vi "main.vi"(8 "error in (no error)":errorcluster, 10 "stages":refnum<class "_stage.lvclass">[](array[class]), 11 "_camera":refnum<class "_camera.lvclass">) -> ()   [LabVIEW 2019]
uses:
  _camera/_camera.lvlibp/_cameraClass/_camera.lvclass
  _stage/_stage.lvlibp/_stageClass/_stage.lvclass
  data_algorithm.ctl
  state.ctl
  data_process.ctl
  <vilib>/Analysis/baseanly.llb/Mean (DBL).vi
  378a35e6-17c3-42fc-973f-4dbb75f37032.vi
  972fad81-3ff3-4c5b-b5d6-c93ea4aec52b.vi
  951adbdd-488d-47b0-b06c-8d69e9ccb4aa.vi
  2b97118a-447f-4295-80f1-8ed8751fa7ac.vi
  <vilib>/Utility/config.llb/Read Key (Path).vi
  <vilib>/Utility/config.llb/Read Key (String).vi
  _camera/_camera.lvlibp/_cameraClass/Write stage positions readback.vi
  _camera/_camera.lvlibp/_cameraClass/Write config file path.vi
  _camera/_camera.lvlibp/_cameraClass/Read camera name and version.vi
  _camera/_camera.lvlibp/_cameraClass/Read wavelength.vi
  _camera/_camera.lvlibp/_cameraClass/Write background.vi
  <vilib>/gmath/NumericalOptimization/Nonlinear Curve Fit LM formula string.vi
  _camera/_camera.lvlibp/_cameraClass/Write wavelength.vi
  _camera/_camera.lvlibp/_cameraClass/Read stage positions.vi
  _camera/_camera.lvlibp/_cameraClass/Write stage positions.vi
  <vilib>/Utility/file.llb/Read Delimited Spreadsheet (DBL).vi
  <vilib>/Utility/config.llb/Read Key (Double).vi
  <vilib>/Analysis/NI_AALBase.lvlib
  <vilib>/Utility/config.llb/NI_LVConfig.lvlib
  <vilib>/gmath/NI_Gmath.lvlib
panel:
  out "signal anis. (accum.)":dbl[][](graph)
  in  "FROG wl_min_max":dbl[](array[numeric])
  out "millisecond timer value 2":u32
  out "Boolean 3":bool=TRUE
  out "cont acq. time":u32
  out "millisecond timer value":u32
  out "plot time":u32
  out "data proc.":u32
  in  "indep?":bool[](array[boolean])
  out "scan done?":bool
  in  "FROG?":bool
  out "size of dependent time scan":i32
  out "single acq. time":u32
  out "single loop time":u32=150 caption="usec"
  in  "which plot":u16(ring)=2 items=["pumped", "unpumped", "reference", "difference"]
  in  "Algorithm":T1=3 items=["<(S*-S)/S>/ln(10)", "<S*/S>-1", "<S*/PD*>/<S/PD>", "<S*/Sref*>/<S/Sref>", "<S*/Sref*/PD*>/<S/Sref>", "<S*/Sref*>/<S/Sref>_alt", "MA/r", "MA/r Sagnac", "FROG"]
  in  "show reference spectrum?":bool
  in  "remove cursor":bool
  in  "add cursor":bool
  out "Array":i32[](array[numeric])
  out "x = y?":bool
  in  "reversed?":bool[](array[boolean])=[TRUE]
  in  "Experimenter":string="who are you?"
  in  "Title":string="A clever title"
  in  "Experimental parameters":string="sample:\nsolvent:\ncuvette:\noptical density:\nexcitation wavelength:\nexcitation power:\nexcitation spot size:\nexcitation fluence: \nprobe spot size:\ncomment:"
  out "current scan":i32
  in  "N scans":u16=5
  in  "sample":string="testSample"
  in  "Experiment":string="testExp"
  in  "center cursor":bool
  in  "save flag":bool
  in  "save type":bool[](array[boolean])=[FALSE, FALSE, FALSE, FALSE]
  in  "data folder":path=path "Z:/11 Setups/04 NOPA TA/01 Data"
  out "progress":dbl(slide)=21.0 scale=0.0..100.0
  out "scan progress":u8(slide)=16 scale=0.0..100.0
  out "Cursor position (wl)":dbl[](array[numeric]) format="%#.2g"
  out "Cursor position (idx)":dbl[](array[numeric])
  in  "ampl":cluster{dbl, dbl}(slide)={-0.2917505030181087, 6.9678068410462775} scale=-1.0..10.0
  in  "diff":dbl(slide)=26.28128772635815 scale=0.05..50.0
  out "main graph":cluster{"wavelength":dbl[], "ref mean":dbl[]}[](graph)
  in  "time delay file":path=path "D:/github/TransientAbsorptionDAQ.lv/stepfiles/01_coarseSteps_-1000_1000fs.txt"
  in  "scan":bool
  in  "bottom panel":u16(ring)=2 items=["x/y", "y/x", "traces", "std", "debug", "debug 2", "parameters", "wavelength"]
  in  "parity?":enum32{"Item 0", "Item 1"}(radio)
  out "Camera initialised?":bool[](array[boolean])
  out "Char":i16
  in  "view error anal":bool
  in  "view full data":bool
  in  "get bg":bool
  in  "cont acq":bool
  in  "move stage":enum32{"Item 0", "Item 1"}(radio)
  out "timed out?":bool
  out "Boolean":bool
  out "Stage(s) initialized":bool[](array[boolean])
  in  "set as t0":bool[](array[boolean])
  in  "home stages":bool[](array[boolean])
  out "stage name(s)":i32[](listbox)
  out "Tab Control":T2(tab)
  out "Intensity Chart":dbl[][](graph)
  out "Intensity Graph":dbl[][](graph)
  out "Waveform Chart":T3(graph)
  out "std graph":cluster{"wavelength":dbl[], "ref std":dbl[]}[](graph)
  out "std":dbl
  out "std":dbl
  out "skipped":bool[](array[boolean])
  out "chopper out":bool[][](array[boolean])
  out "synchronization error":bool
  out "mean":dbl
  out "mean":dbl
  out "PD hist":T4(graph)
  out "PD":cluster{i32[], dbl[]}[](graph)
  in  "ts_plot_lin-log":bool caption="timestep_plot_linlog"
  out "base path":path
  out "stage config":path
  out "camera config":path
  out "Application Directory":path
  out "appended path":path
  out "Stage objects":refnum<class "_stage.lvclass">[](array[class])
  out "timesteps loaded from file":dbl[][](array[numeric])
  out "size of dependent time scan 2":i32
  out "Waveform Graph":dbl[](graph)
  in  "trig2 level":dbl(slide)=783.9195979899498 scale=0.0..2000.0
  out "Tank 2":dbl(slide) scale=0.0..2000.0
  out "Tank 2 + std":dbl(slide) scale=0.0..2000.0
  out "Tank 2 - std":dbl(slide) scale=0.0..2000.0
  in  "trig1 level":dbl(slide)=783.9195979899498 scale=0.0..2000.0
  out "Tank 1":dbl(slide)=552.7638190954774 scale=0.0..2000.0
  out "Tank 1 - std":dbl(slide) scale=0.0..2000.0
  out "Tank 1 + std":dbl(slide) scale=0.0..2000.0
  in  "baseline offset (ref.)":dbl
  in  "baseline offset (signal)":dbl
  in  "history length":i32=20
  in  "Scale.Range:Maximum":dbl(slide)=43.976036093027226 caption="diff scale range" scale=1.0..1000.0
  in  "camera max scale":u16(ring) items=["16-bit", "14-bit", "12-bit"]
  in  "save raw data":bool caption="saw raw data"
  in  "is measurement TA?":bool=TRUE
  out "Boolean 2":bool
  out "element 2":dbl
  out "element 3":dbl
  out "PDs mean":dbl[](array[numeric])
  out "PDs std":dbl[](array[numeric])
  out "dynamic offset":dbl[](array[numeric])
  in  "use dynamic offset?":bool
  in  "save wl calibration to .ini":bool caption="calibrate_wl"
  in  "index":u16
  in  "calibrate wavelength":bool caption="calibrate_wl"
  out "wavelength fit":cluster{i32[], dbl[]}[](graph)
  out "wavelength (fitted)":dbl[](array[numeric]) format="%#.0f"
  in  "wavelength \n(calibration value)":dbl[](array[numeric]) caption="wavelength (calibration value)"
  in  "pixel/index":u16[](array[numeric])
  in  "mirror?":bool
  in  "initial parameters":dbl[](array[numeric])=[150.0, 200000.0, 1200.0]
  out "best fit parameters":dbl[](array[numeric])
  in  "t0 position(s)":dbl[](array[numeric]) caption="t0 (s)" format="%07.0f"
  out "stage position(s) readback":dbl[](array[numeric]) caption="readback (fs)" format="%09.1f"
  in  "stage position(s)":dbl[](array[numeric]) caption="set (fs)" format="%09.1f"
  out "camera name, version":string
  in  "get_single_acq":bool caption="get single"
  out "vi running?":bool=TRUE
  out "is moving?":bool[](array[boolean]) caption="mov?"
  # "scan"
  # "out of"
  # "just temp ..."
  # "timing"
  # "usec"
  # "transient"
  # "pumped mean"
  # "unpumped mean"
  # "reference mean"
  # "Hartmann dispersion formula:"
  # "d(\\lambda) = a1 + a2 / (pix - a3)"
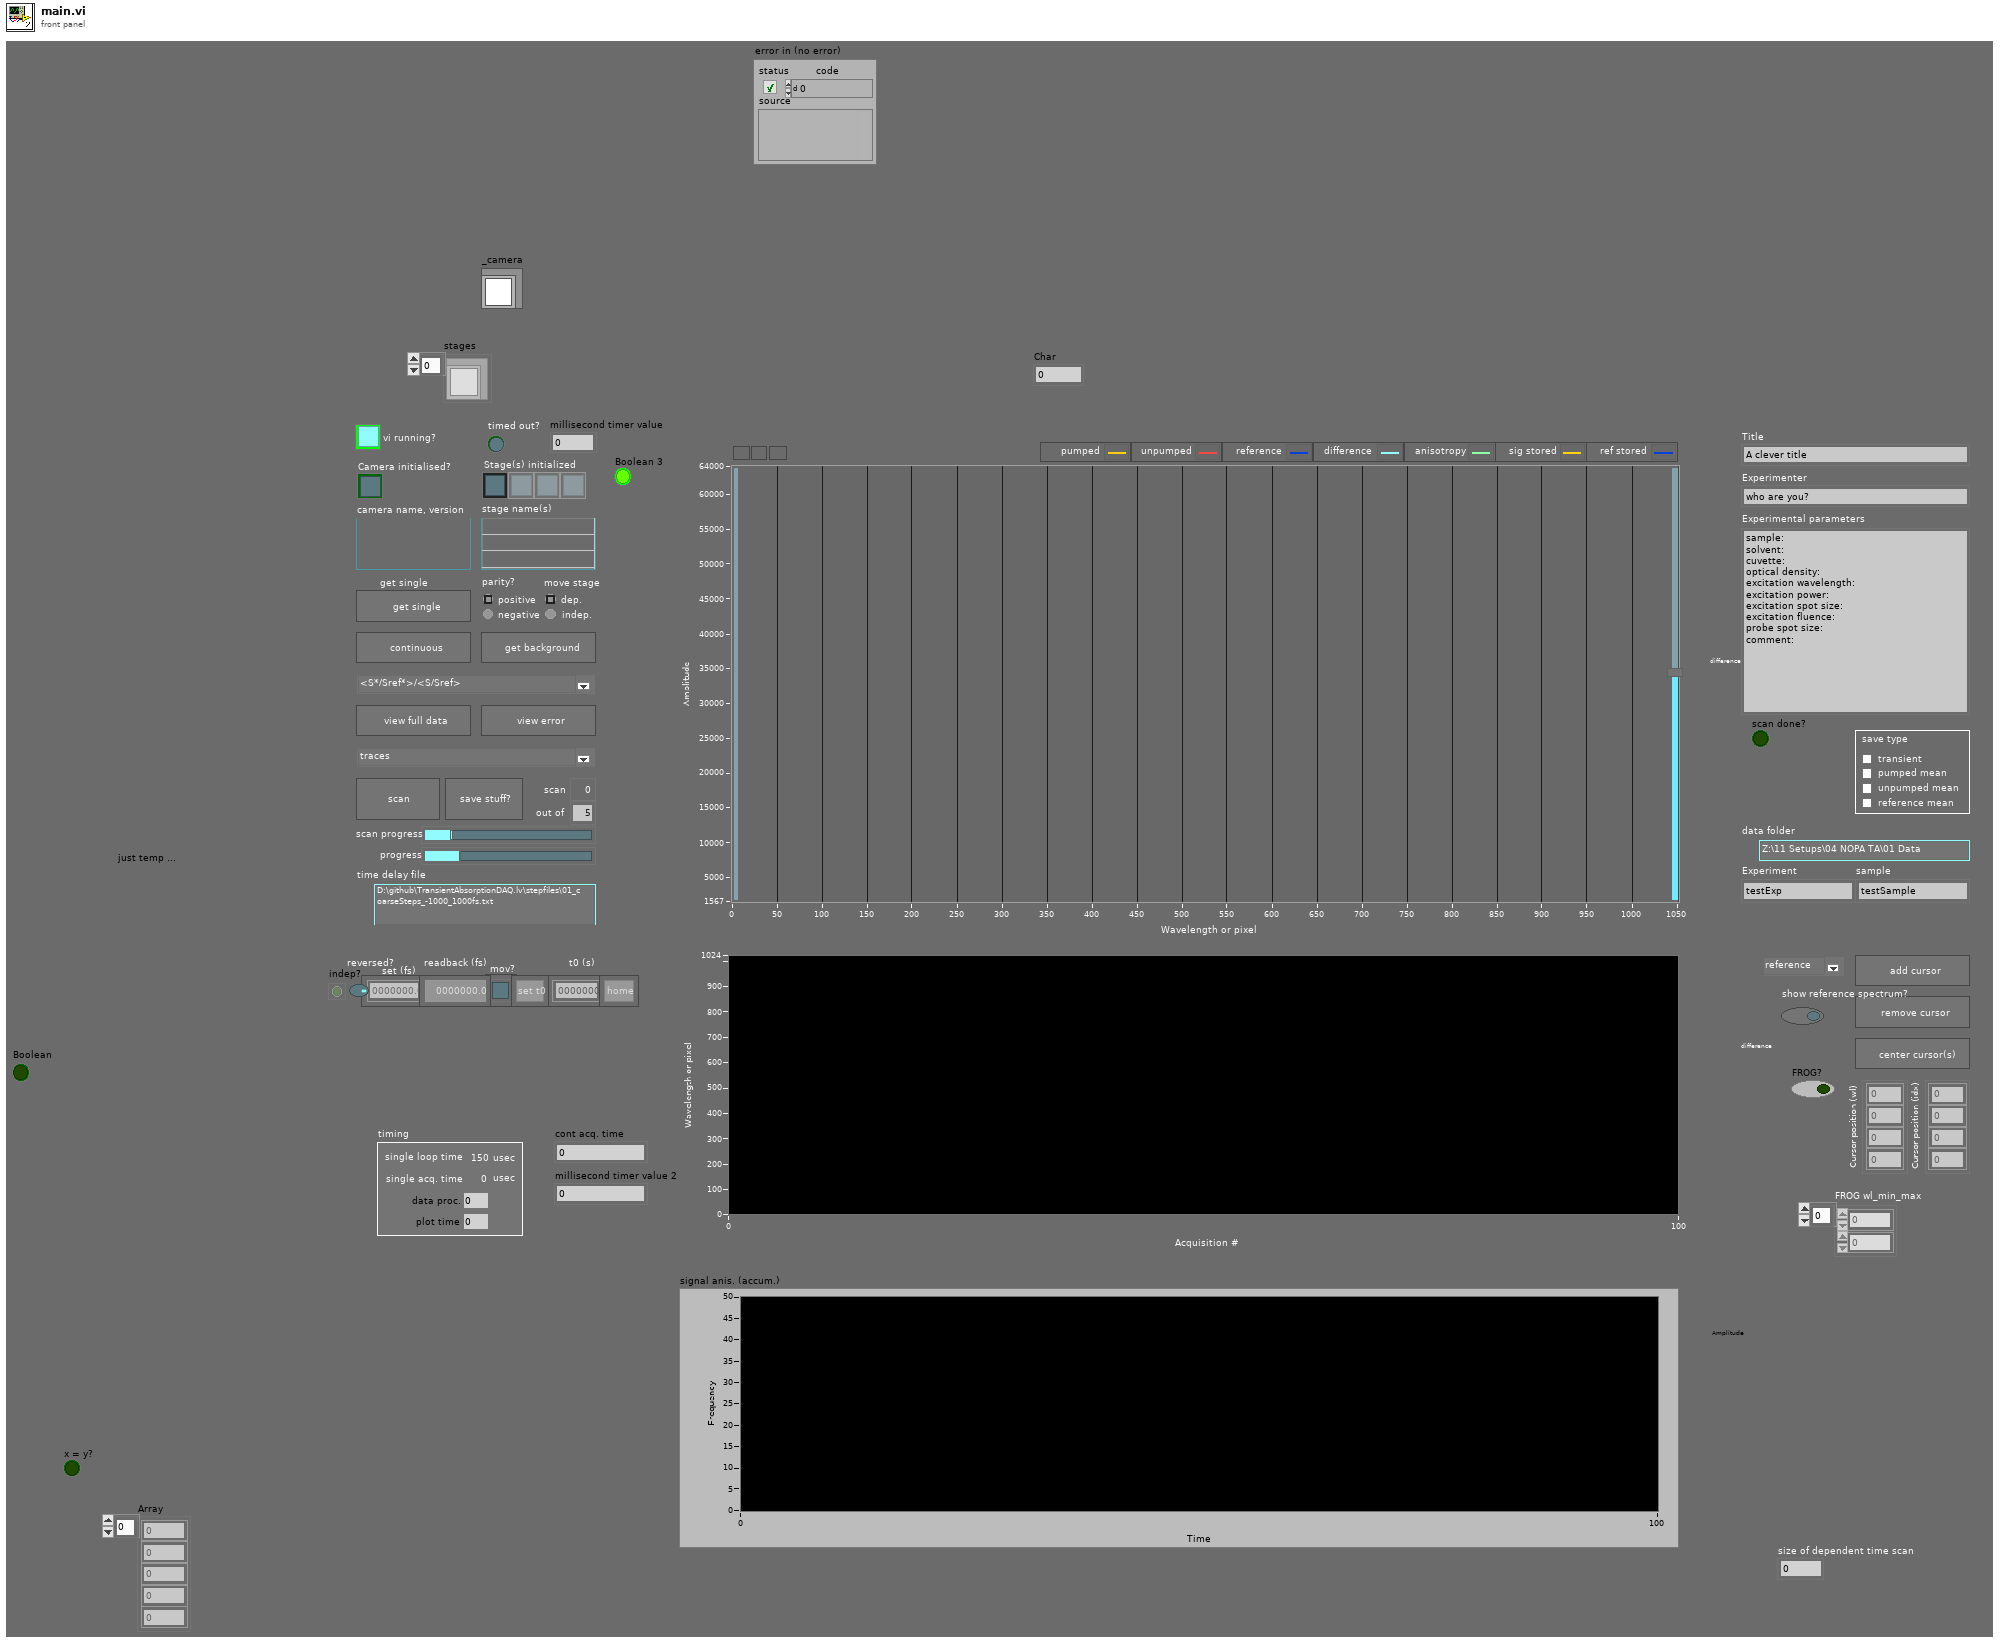
[diagram p1: front panel]
types:
  T1 = typedef "data_algorithm.ctl" = u16
  T2 = enum32{"x/y", "y/x", "traces", "std", "debug", "debug 2", "parameters", "wavelength"}
  T3 = cluster{"[0]":dbl, "[1]":dbl, "[2]":dbl, "[3]":dbl, "[4]":dbl, "[5]":dbl, "[6]":dbl, "[7]":dbl, "[8]":dbl}
  T4 = cluster{"Histogram: h(x)":i32[], "X Values":dbl[]}[]
  T5 = typedef "data_process.ctl" = enum16{"timeout", "init", "reset", "process", "plot", "post-processing", "save", "exit"}
  T6 = cluster{"type":string, "raw data":dbl[][][], "wavelength":dbl[], "trigger":bool[][], "stage position (set) [fs]":dbl[], "stage position (readback) [fs]":dbl[], "scn_step_pos (set)":dbl[], "scn_step_time_dly (set) [fs]":dbl[][], "scn_step":i32, "scn_iter":i32, "command":T5, "save flag":bool, "save path":path, "save type":bool[], "raw PDs":dbl[][], "scan done?":bool}
  T7 = typedef "state.ctl" = enum16{"timeout", "hw_init", "sw_init", "cam_single_acq", "cam_get_bg", "cam_rst_bg", "cam_cnt_acq", "cam_set_wl", "stg_set_pos", "stg_home", "scn_load_step_file", "scn_init", "scn_next_step", "scn_next_iter", "dat_update_save_flag", "dat_update_save_type", "dat_save_raw", "dat_send_to_process", "aux_save_wl_to_ini", "aux_center_cursor", "stop"}
  T8 = cluster{"acq num":u32[], "curr acq":i32, "signal":dbl[], "signal anis.":dbl[], "signal (accum.)":dbl[][], "signal anis. (accum.)":dbl[][], "pumped mean":dbl[], "unpumped mean":dbl[], "reference mean":dbl[], "pumped std":dbl[], "unpumped std":dbl[], "reference std":dbl[], "pumped stored":dbl[], "reference stored":dbl[], "signal std":dbl[]}
  T9 = typedef "NI_LVConfig.lvlib/Config Data RefNum.ctl" = refnum<k1>
  T10 = enum32{"invalid app kind", "Development System", "Run Time System", "Student Edition", "Embedded LabVIEW", "Evaluation", "Custom"}
  T11 = cluster{"model":string, "Parameters":string[], "x":string}
  T12 = typedef "LVRangeTypeDef.ctl" = cluster{"Minimum":dbl, "Maximum":dbl, "Increment":dbl, "Minor Increment":dbl, "Start":dbl}
  T13 = typedef "LVCursorListTypeDef.ctl" = cluster{"Name":string, "Color":u32, "Style":u8, "Point Style":u8, "Name Visible":bool, "Allow Drag":bool, "Cursor Mode":u32, "Plot":i32, "Index":i32, "Position":cluster{"X":dbl, "Y":dbl}, "X Scale":u32, "Y Scale":u32, "Watch Plots":i32[], "Watch All Plots":bool, "Plot Area":i32, "Label Offset":cluster{"X":dbl, "Y":dbl}}[]
  T14 = cluster{"Name":string, "Color":u32, "Style":u8, "Point Style":u8, "Name Visible":bool, "Allow Drag":bool, "Cursor Mode":u32, "Plot":i32, "Index":i32, "Position":cluster{"X":dbl, "Y":dbl}, "X Scale":u32, "Y Scale":u32, "Watch Plots":i32[], "Watch All Plots":bool, "Plot Area":i32, "Label Offset":cluster{"X":dbl, "Y":dbl}}
  T15 = cluster{"wavelength":dbl[], "unpumped mean":dbl[]}
  T16 = cluster{"wavelength":dbl[], "reference mean":dbl[]}
  T17 = cluster{"wavelength":dbl[], "reference stored":dbl[]}
  T18 = cluster{"wavelength":dbl[], "pumped stored":dbl[]}
  T19 = cluster{"wavelength":dbl[], "signal anis.":dbl[]}
  T20 = cluster{"Histogram: h(x)":i32[], "X Values":dbl[]}
  T21 = cluster{"wavelength":dbl[], "reference stored":dbl[]}[]
  T22 = cluster{"wavelength":dbl[], "unpumped std":dbl[]}
  T23 = cluster{"wavelength":dbl[], "reference std":dbl[]}
  T24 = cluster{"wavelength":dbl[], "reference std":dbl[]}[]
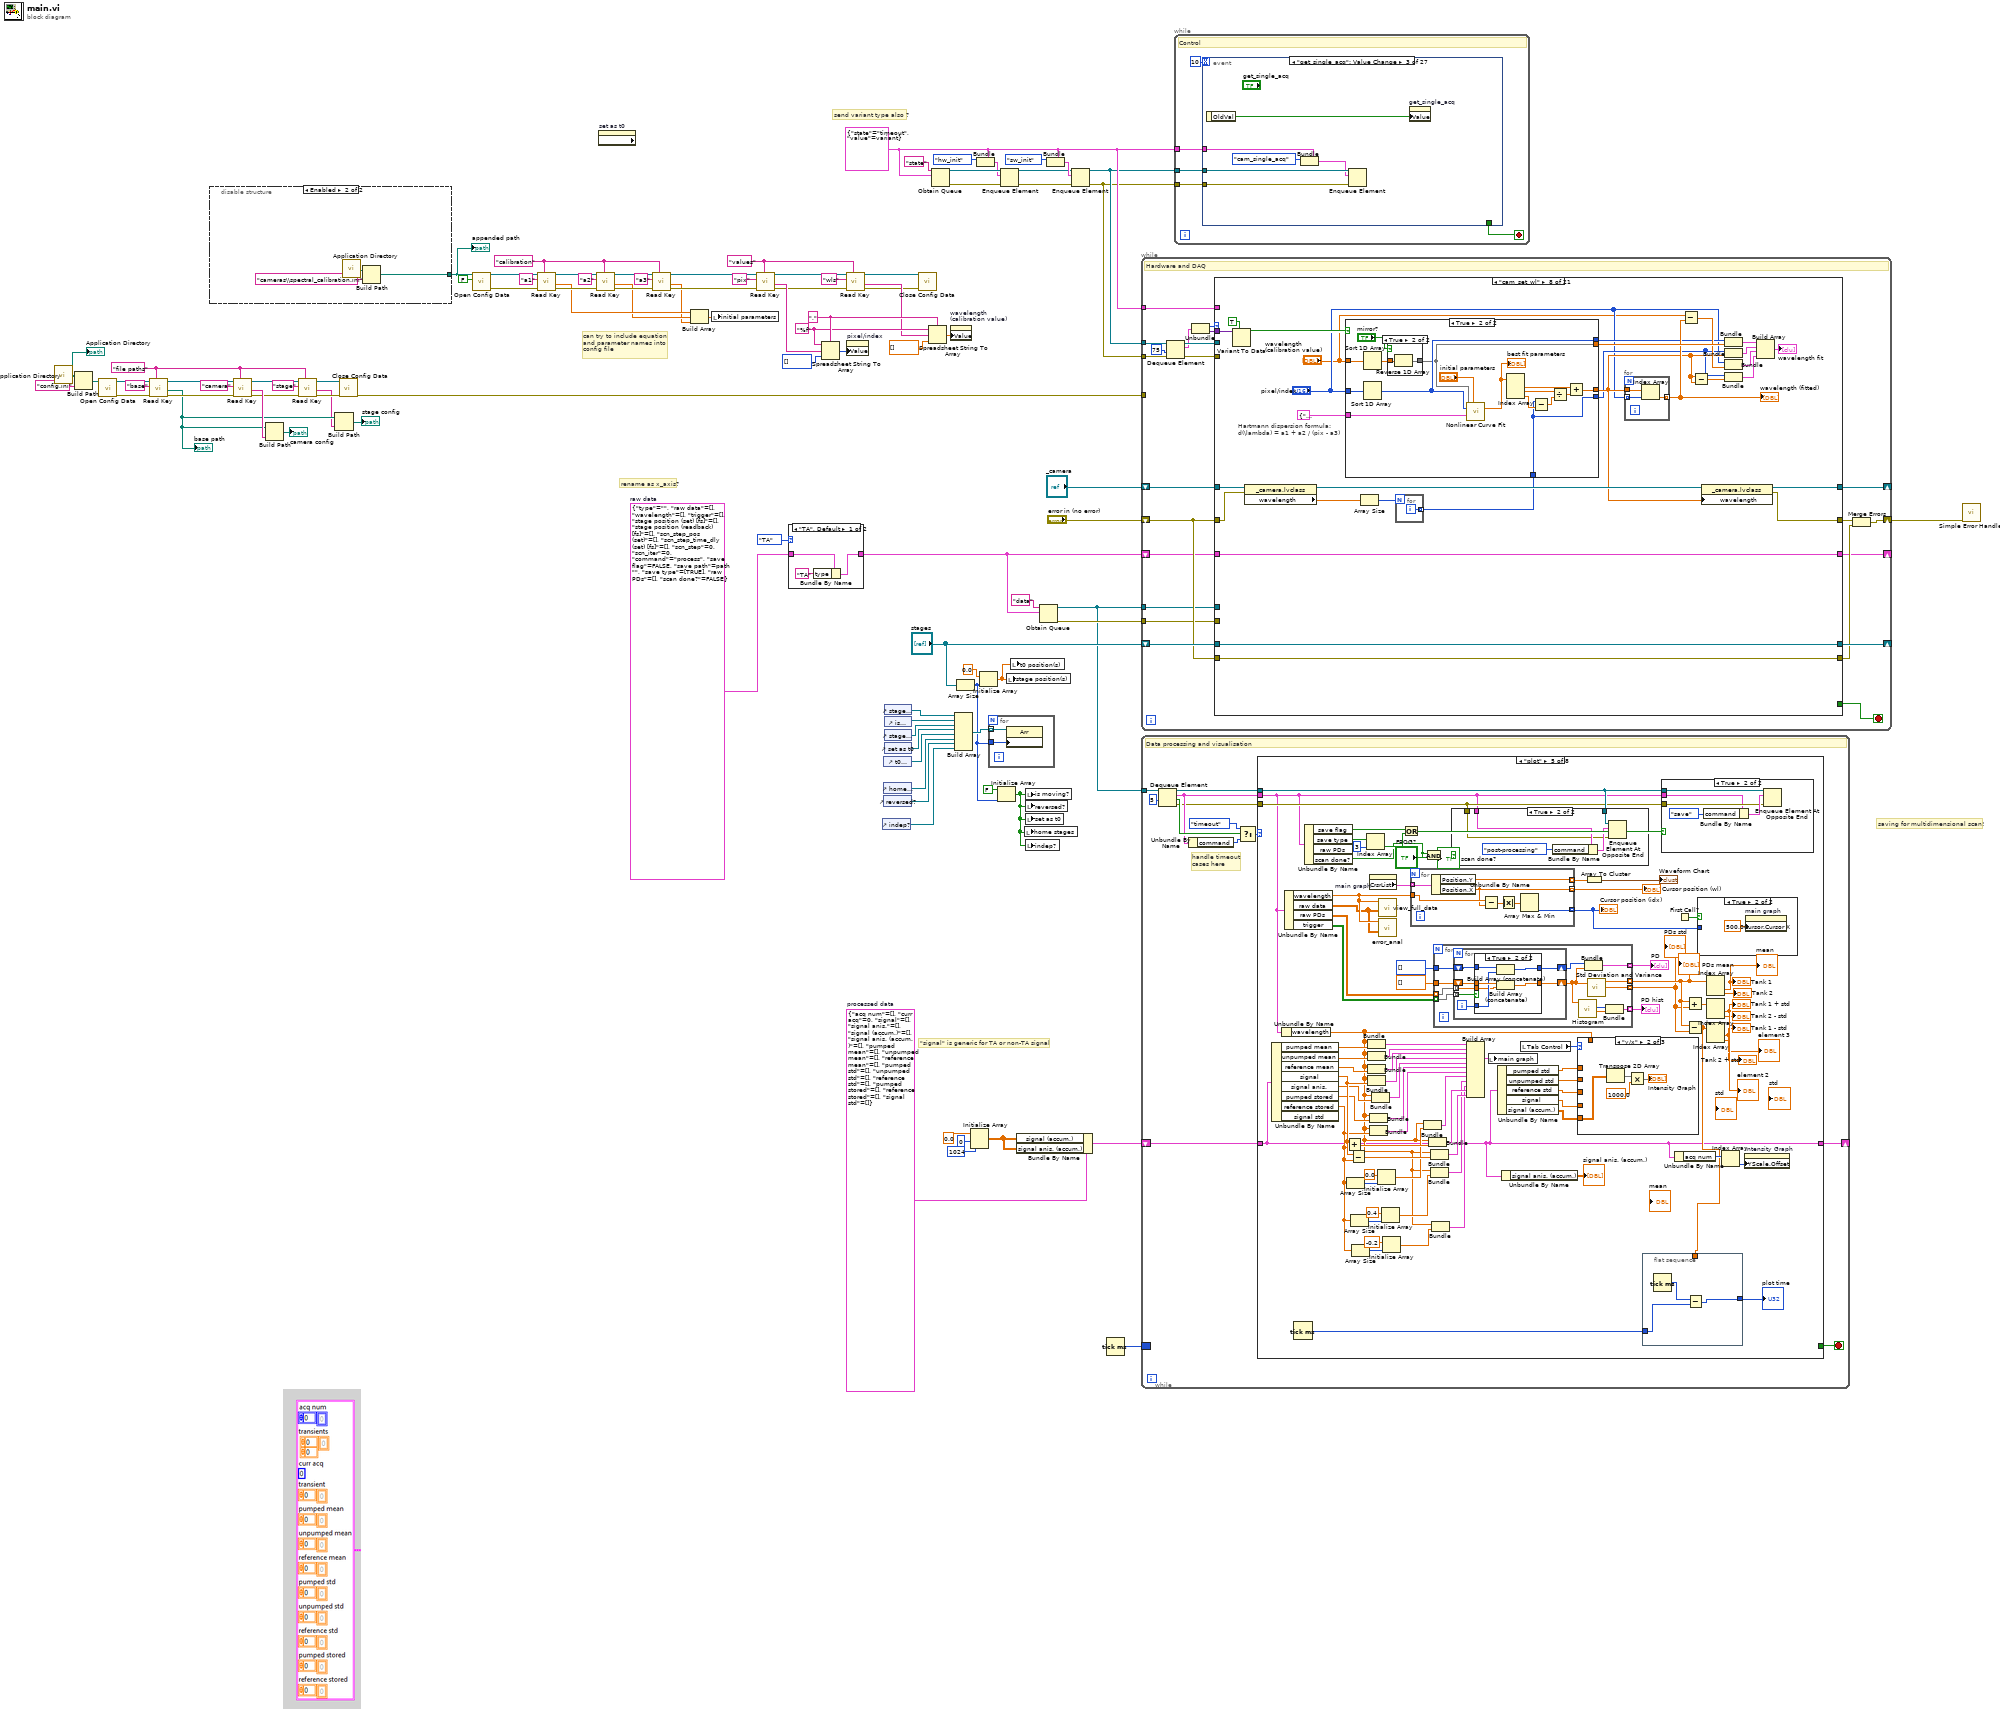
[diagram p0: block diagram]
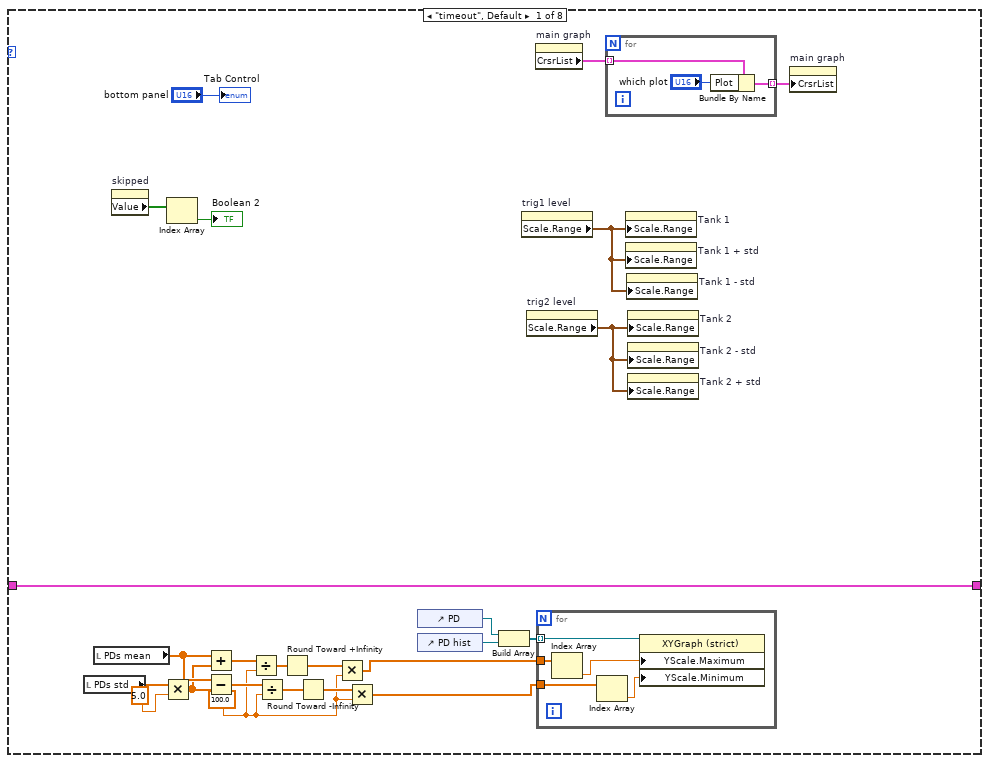
[diagram p2: hidden frame]
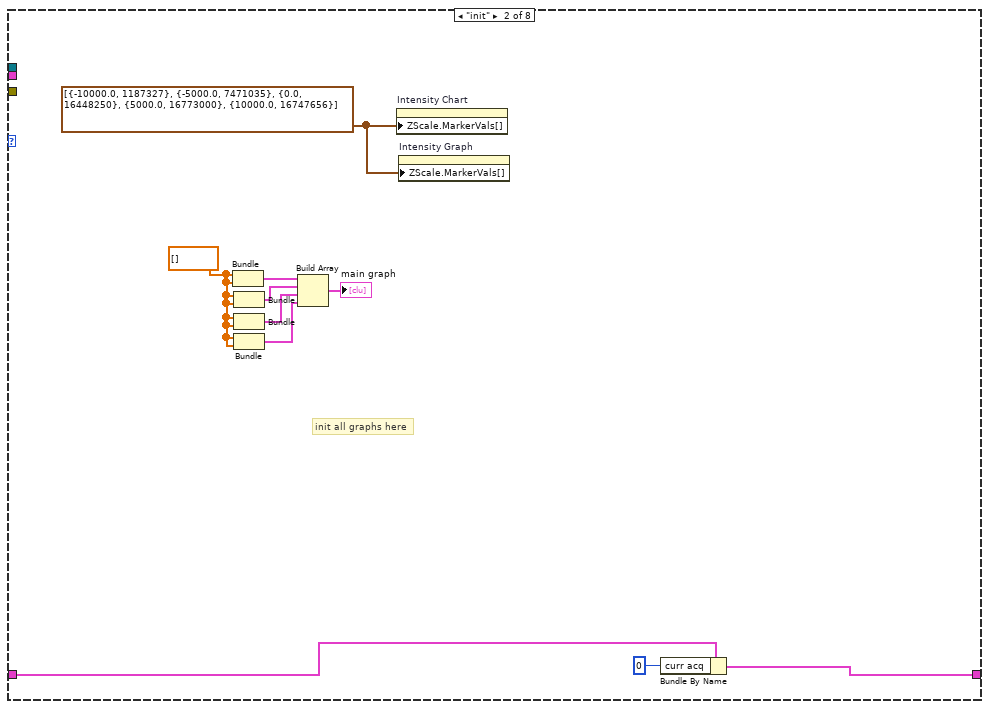
[diagram p3: hidden frame]
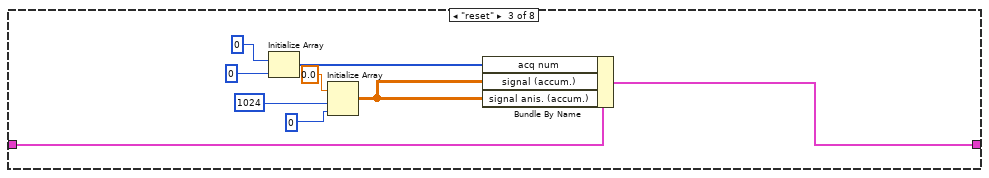
[diagram p4: hidden frame]
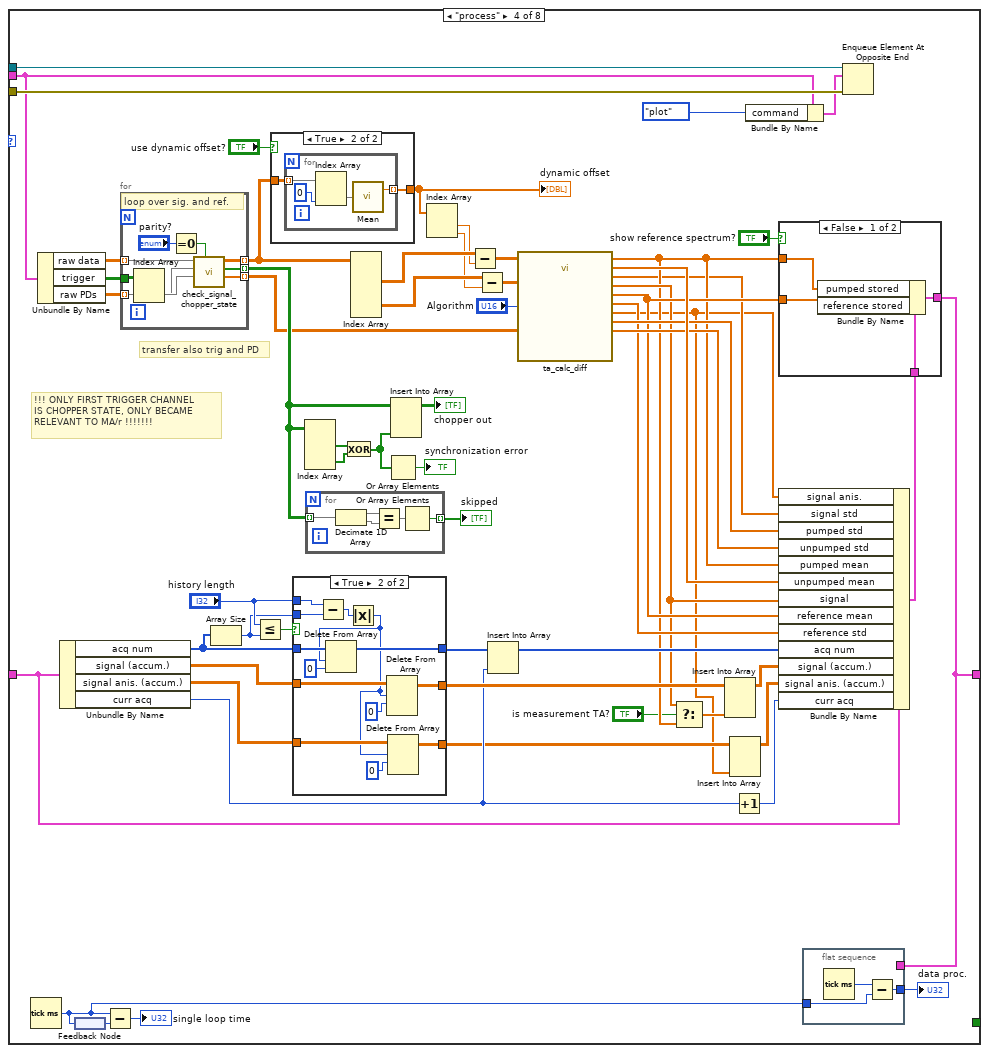
[diagram p5: hidden frame]
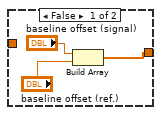
[diagram p6: hidden frame]
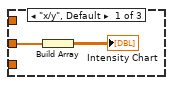
[diagram p13: hidden frame]
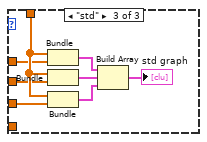
[diagram p14: hidden frame]
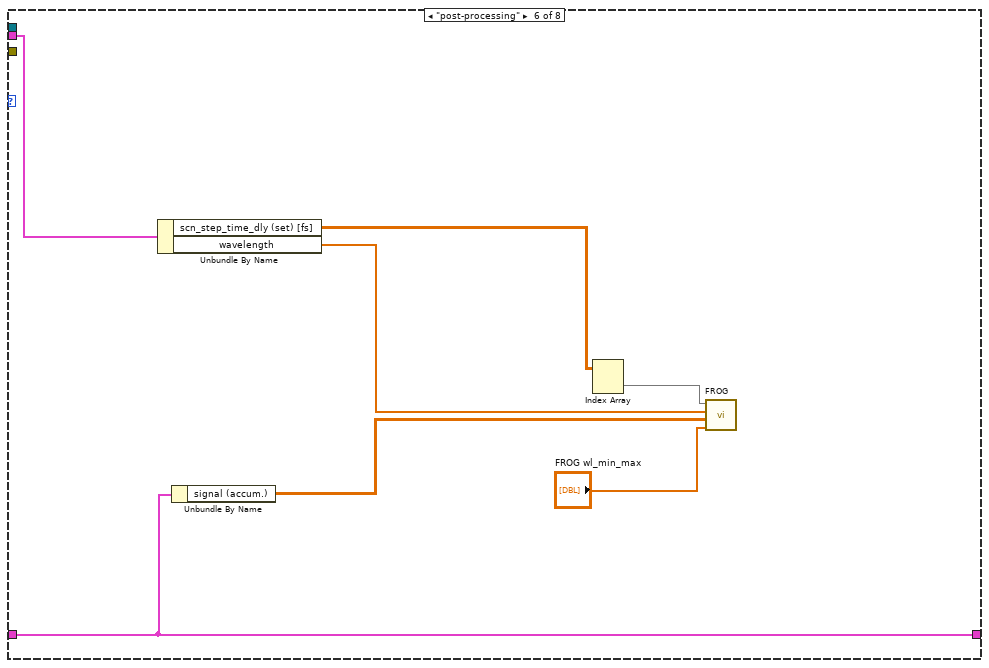
[diagram p15: hidden frame]
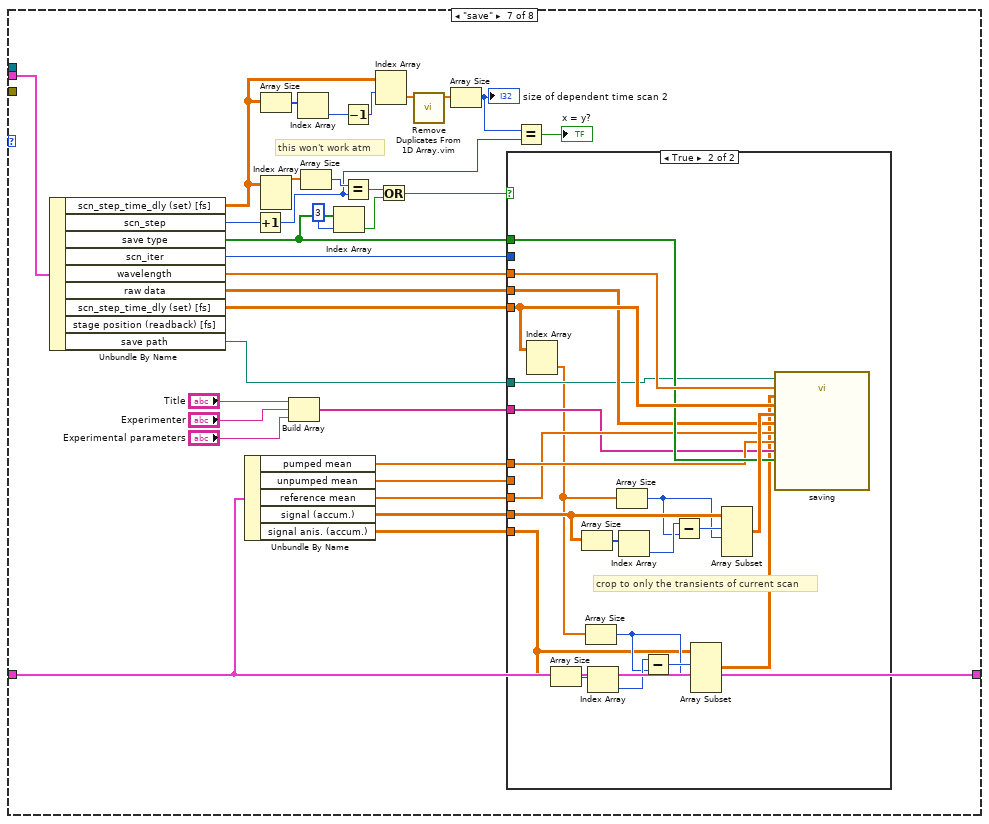
[diagram p16: hidden frame]
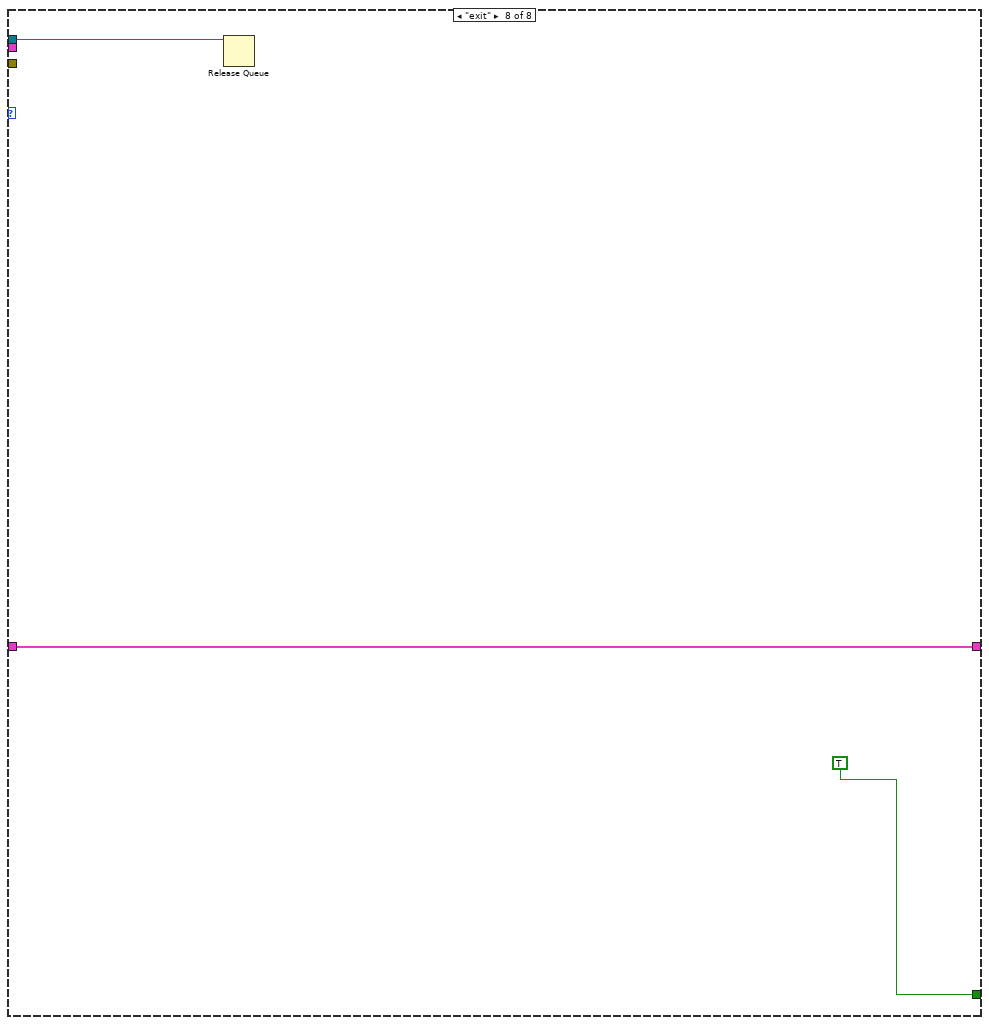
[diagram p18: hidden frame]
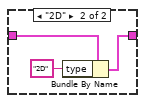
[diagram p19: hidden frame]
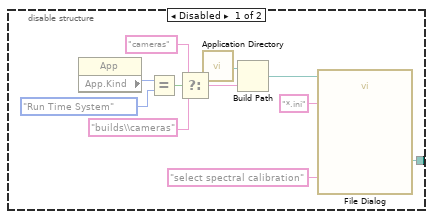
[diagram p20: hidden frame]
diagram:
  w14 = "," ("delimiter (Tab)")
  w13 = "%f" ("format string")
  w15 = "values" ("section")
  w29 = "calibration" ("section")
  w37 = T6 {"type"="", "raw data"=[], "wavelength"=[], "trigger"=[], "stage position (set) [fs]"=[], "stage position (readback) [fs]"=[], "scn_step_pos (set)"=[], "scn_step_time_dly (set) [fs]"=[], "scn_step"=0, "scn_iter"=0, "command"=enum."process", "save flag"=FALSE, "save path"=path "", "save type"=[TRUE], "raw PDs"=[], "scan done?"=FALSE}  # raw data
  w41 = "file paths" ("section")
  w36 = T8 {"acq num"=[], "curr acq"=0, "signal"=[], "signal anis."=[], "signal (accum.)"=[], "signal anis. (accum.)"=[], "pumped mean"=[], "unpumped mean"=[], "reference mean"=[], "pumped std"=[], "unpumped std"=[], "reference std"=[], "pumped stored"=[], "reference stored"=[], "signal std"=[]}  # processed data
  w63 = cluster{"state":T7, "value":variant} {"state"=enum."timeout", "value"=variant}
  # "can try to include equation\nand parameter names into \nconfig file"
  # "saving for multidimensional scan!"
  # "\"signal\" is generic for TA or non-TA signal"
  # "rename as x_axis?"
  # "send variant type also ?"
  n1 = call <vilib>:"Application Directory.vi"() -> ("Application Directory"=w56:path)
  "Application Directory" <- w56
  n2 = Build Path(base path=w56, name or relative path="config.ini") -> (appended path=w54:path)
  n3 = call <vilib>:"Open Config Data.vi"("configuration file path"=w54) -> ("error out"=w58:errorcluster, "refnum"=w59:T9)  [unwired: 8 in, 1 out]
  n4 = call-poly <vilib>:"Read Key.vi"("section"=w41, "error in (no error)"=w58, "key"="base", "refnum"=w59) -> ("error out"=w48:errorcluster, "value"=w46:path, "refnum out"=w49:T9)  [unwired: 4 in, 1 out]
  "base path" <- w46
  n5 = disable-structure shown="Enabled" {
    disable-tunnel: [w108 w109] -> w68
    frame Disabled {
      n6 = property class="App"() -> ("App.Kind"=w105:T10)  [unwired: 2 in, 2 out]
      n7 = Equal?(x=w105, y=T10."Run Time System") -> (x = y?=w103:bool)
      n8 = Select(t="cameras" ("name or relative path"), s=w103, f="builds\\cameras" ("name or relative path")) -> (s? t:f=w100:string)
      n9 = call <vilib>:"Application Directory.vi"() -> ("Application Directory"=w107:path)
      n10 = Build Path(base path=w107, name or relative path=w100) -> (appended path=w106:path)
      n11 = call "File Dialog"("start path"=w106, "prompt"="select spectral calibration", "pattern (all files)"="*.ini") -> ("selected path"=w108:path)  [unwired: 9 in, 3 out]
    }
    frame Enabled {
      n12 = call <vilib>:"Application Directory.vi"() -> ("Application Directory"=w111:path)
      n13 = Build Path(base path=w111, name or relative path="cameras\\spectral_calibration.ini") -> (appended path=w109:path)
    }
  }
  "appended path" <- w68
  n14 = call-poly <vilib>:"Read Key.vi"("section"=w41, "error in (no error)"=w48, "key"="camera", "refnum"=w49) -> ("error out"=w43:errorcluster, "value"=w47:string, "refnum out"=w42:T9)  [unwired: 4 in, 1 out]
  n15 = Build Path(base path=w46, name or relative path=w47) -> (appended path=→"camera config":path)
  n16 = call-poly <vilib>:"Read Key.vi"("section"=w41, "error in (no error)"=w43, "key"="stage", "refnum"=w42) -> ("error out"=w51:errorcluster, "value"=w45:string, "refnum out"=w52:T9)  [unwired: 4 in, 1 out]
  n17 = Build Path(base path=w46, name or relative path=w45) -> (appended path=→"stage config":path)
  n18 = call <vilib>:"Close Config Data.vi"("error in (no error)"=w51, "refnum"=w52) -> ("error out"=w39:errorcluster)  [unwired: 8 in, 1 out]
  n19 = call <vilib>:"Open Config Data.vi"("create file if necessary (T)"=FALSE, "configuration file path"=w68) -> ("error out"=w33:errorcluster, "refnum"=w34:T9)  [unwired: 7 in, 1 out]
  n20 = call-poly <vilib>:"Read Key.vi"("section"=w29, "error in (no error)"=w33, "key"="a1", "refnum"=w34) -> ("error out"=w27:errorcluster, "value"=w7:dbl, "refnum out"=w28:T9)  [unwired: 4 in, 1 out]
  n21 = call-poly <vilib>:"Read Key.vi"("section"=w29, "error in (no error)"=w27, "key"="a2", "refnum"=w28) -> ("error out"=w26:errorcluster, "value"=w6:dbl, "refnum out"=w25:T9)  [unwired: 4 in, 1 out]
  n22 = property on="set as t0" class="Arr" props=["Number of Rows"]() -> ()  [unwired: 2 in, 3 out]
  n23 = call-poly <vilib>:"Read Key.vi"("section"=w29, "error in (no error)"=w26, "key"="a3", "refnum"=w25) -> ("error out"=w23:errorcluster, "value"=w5:dbl, "refnum out"=w24:T9)  [unwired: 4 in, 1 out]
  n24 = Build Array(w7, w6, w5) -> (w4:dbl[])
  n25 = local write "initial parameters"(w4) -> ()
  n26 = call-poly <vilib>:"Read Key.vi"("section"=w15, "error in (no error)"=w23, "key"="pix", "refnum"=w24) -> ("error out"=w16:errorcluster, "value"=w22:string, "refnum out"=w17:T9)  [unwired: 4 in, 1 out]
  n27 = case shown="\"TA\", Default" enum16{"TA", "2D"}."TA" {
    tunnel: [w112 w116] -> w70
    tunnel: w37 -> [w114 w117]
    frame "TA", Default {
      n28 = Bundle By Name(cluster=w114, "type"="TA") -> (w112:T6)
    }
    frame "2D" {
      n29 = Bundle By Name(cluster=w117, "type"="2D") -> (w116:T6)
    }
  }
  n30 = Spreadsheet String To Array(delimiter (Tab)=w14, format string=w13, spreadsheet string=w22, array type (2D Dbl)=i32[] []) -> (array=w19:i32[])
  n31 = call-poly <vilib>:"Read Key.vi"("section"=w15, "error in (no error)"=w16, "key"="wls", "refnum"=w17) -> ("error out"=w8:errorcluster, "value"=w12:string, "refnum out"=w9:T9)  [unwired: 4 in, 1 out]
  n32 = property on="pixel/index" class="Arr (strict)"("Value"=w19) -> ()  [unwired: 2 in, 2 out]
  n33 = control-ref of="indep?"() -> (w2:refnum<vi>)
  n34 = control-ref of="t0 position(s)"() -> (w83:refnum<vi>)
  n35 = control-ref of="home stages"() -> (w82:refnum<vi>)
  n36 = control-ref of="reversed?"() -> (w60:refnum<vi>)
  n37 = control-ref of="stage position(s)"() -> (w85:refnum<vi>)
  n38 = control-ref of="is moving?"() -> (w88:refnum<vi>)
  n39 = control-ref of="stage position(s) readback"() -> (w87:refnum<vi>)
  n40 = control-ref of="set as t0"() -> (w84:refnum<vi>)
  n41 = call <vilib>:"Close Config Data.vi"("error in (no error)"=w8, "refnum"=w9) -> ()  [unwired: 8 in, 2 out]
  n42 = Spreadsheet String To Array(delimiter (Tab)=w14, format string=w13, spreadsheet string=w12, array type (2D Dbl)=dbl[] []) -> (array=w10:dbl[])
  n43 = Obtain Queue(name (unnamed)="state", element data type=w63) -> (queue out=w95:refnum<queue>, error out=w94:errorcluster)  [unwired: 3 in, 1 out]
  n44 = property on="wavelength \n(calibration value)" class="Arr (strict)"("Value"=w10) -> ()  [unwired: 2 in, 2 out]
  n45 = Build Array(w85, w88, w87, w84, w83, w82, w60, w2) -> (w86:refnum<vi>[])
  n46 = Array Size(array="stages") -> (size(s)=w79:i32)
  n47 = Initialize Array(0.0, 0 ("dimension size"), 1024 ("dimension size")) -> (w1:dbl[][])
  n48 = Bundle(cluster=w63, "state"=state."hw_init") -> (w81:cluster{"state":T7, "value":variant})  [unwired: 1 in]
  n49 = Initialize Array(0.0, w79) -> (w78:dbl[])
  n50 = for {
    tunnel: w86 -> [w118] mode=indexing
    tunnel: w79 -> [w119]
    n51 = property class="Arr"(reference=w118, "Number of Rows"=w119) -> ()  [unwired: 1 in, 2 out]
  }
  n52 = Initialize Array(FALSE, w79) -> (w3:bool[])
  n53 = Enqueue Element(queue=w95, element=w81, error in (no error)=w94) -> (queue out=w65:refnum<queue>, error out=w64:errorcluster)  [unwired: 1 in, 1 out]
  n54 = local write "stage position(s)"(w78) -> ()
  n55 = local write "t0 position(s)"(w78) -> ()
  n56 = Bundle By Name(cluster=w36, "signal (accum.)"=w1, "signal anis. (accum.)"=w1) -> (w74:T8)
  n57 = local write "home stages"(w3) -> ()
  n58 = local write "is moving?"(w3) -> ()
  n59 = local write "reversed?"(w3) -> ()
  n60 = local write "set as t0"(w3) -> ()
  n61 = local write "indep?"(w3) -> ()
  n62 = Obtain Queue(name (unnamed)="data", element data type=w70) -> (queue out=w69:refnum<queue>, error out=w71:errorcluster)  [unwired: 3 in, 1 out]
  n63 = Bundle(cluster=w63, "state"=state."sw_init") -> (w67:cluster{"state":T7, "value":variant})  [unwired: 1 in]
  n64 = Enqueue Element(queue=w65, element=w67, error in (no error)=w64) -> (queue out=w62:refnum<queue>, error out=w61:errorcluster)  [unwired: 1 in, 1 out]
  n65 = Tick Count (ms)() -> (millisecond timer value=w89:u32)
  n66 = while {
    shift-right: [w140] -> _
    shift-left: "_camera" -> [w141]
    tunnel: w62 -> [w120]
    tunnel: w61 -> [w139]
    shift-right: [w131] -> w93
    shift-left: "error in (no error)" -> [w133]
    shift-right: [w135] -> _
    shift-left: "stages" -> [w134]
    tunnel: w63 -> [w125]
    shift-right: [w123] -> _
    shift-left: w70 -> [w129]
    tunnel: w69 -> [w122]
    tunnel: w71 -> [w121]
    tunnel: w39 -> [_]
    stop <- w138 stop-if-true
    # "Hardware and DAQ"
    n67 = Dequeue Element(queue=w120, timeout in ms (-1)=75, error in (no error)=w139) -> (queue out=w137:refnum<queue>, element=w127:cluster{"state":T7, "value":variant}, error out=w136:errorcluster)  [unwired: 1 out]
    n68 = Unbundle(w127) -> ("state"=w126:T7, "value"=w124:variant)
    n69 = case shown="\"cam_set_wl\"" w126 {
      tunnel: w141 -> [w149 w246 w307 w328 w395 w409 w425 w453 w497 w536 w562 w591 w635 w690 w725 w739 w756 w782 w795 w801 w827]
      tunnel: [w148 w259 w307 w325 w393 w408 w425 w458 w501 w536 w562 w591 w635 w690 w725 w739 w756 w782 w795 w801 w826] -> w140
      tunnel: [_ _ _ _ _ _ _ _ _ _ _ _ _ _ _ _ _ _ _ _ w828] -> w138
      tunnel: w137 -> [w155 w227 w301 w318 _ _ w429 _ _ _ _ w586 w631 w693 _ _ w769 _ _ _ w815]
      tunnel: w136 -> [w154 w228 w300 w319 _ _ w428 _ _ _ _ w585 w630 w692 _ _ w768 _ _ _ w814]
      tunnel: w133 -> [w157 w245 w306 w327 w390 w406 w424 w452 w502 w535 w561 w590 w634 w689 w726 w738 w755 w781 w793 w800 w824]
      tunnel: [w156 w257 w306 w324 w384 w405 w424 w457 w502 w535 w561 w590 w634 w689 w726 w738 w755 w781 w793 w800 w822] -> w132
      tunnel: [w150 w238 w305 w320 w388 w404 w423 w456 w494 w534 w548 w589 w632 w688 w728 w734 w752 w780 w791 w798 w818] -> w135
      tunnel: w134 -> [w153 w255 w305 w323 w388 w404 w423 w456 w485 w534 w548 w589 w632 w688 w728 w734 w752 w780 w791 w798 w821]
      tunnel: w133 -> [w152 w252 w304 w322 w387 w403 w422 w455 w491 w533 w560 w588 w633 w687 w727 w733 w751 w779 w792 w797 w820]
      tunnel: [w151 w237 w304 w321 w387 w403 w422 w455 w493 w533 w560 w588 w633 w687 w727 w733 w751 w779 w792 w797 w819] -> w130
      tunnel: w129 -> [w142 w253 w296 w326 w386 w402 w412 w454 w499 w532 w555 w583 w628 w686 w730 w737 w750 w772 w794 w799 w823]
      tunnel: w125 -> [w147 w229 w297 w317 _ _ w415 _ _ _ _ w584 w629 w691 _ _ w759 _ _ _ w809]
      tunnel: w124 -> [w146 _ _ _ _ _ _ w446 w500 _ w559 _ _ _ w724 w735 _ w778 _ _ _]
      tunnel: [w142 w232 w296 w314 w386 w402 w412 w454 w499 w532 w554 w581 w614 w680 w729 w736 w749 w772 w794 w799 w805] -> w123
      tunnel: w122 -> [_ _ _ _ _ _ _ _ _ _ _ _ _ _ _ _ _ w774 _ _ w807]
      tunnel: w121 -> [_ _ _ _ _ _ _ _ _ _ _ _ _ _ _ _ _ w773 _ _ w806]
      frame "timeout", Default {
        w144 = TRUE ("Boolean 2")
        n70 = case shown="No Error" w157 {
          selector: w157 -> [w161 w223]
          tunnel: [w172 w223] -> w156
          tunnel: w155 -> [_ w225]
          tunnel: w154 -> [_ w224]
          tunnel: w153 -> [w169 w221]
          tunnel: w152 -> [w171 w220]
          tunnel: [w170 w220] -> w151
          tunnel: [w168 w221] -> w150
          tunnel: w149 -> [w160 w222]
          tunnel: [w173 w222] -> w148
          tunnel: w147 -> [_ w219]
          tunnel: w146 -> [_ _]
          tunnel: [FALSE TRUE ("Boolean")] -> w145
          tunnel: w144 -> [w166 w213]
          tunnel: [w165 w212] -> w143
          frame No Error {
            n71 = First Call?() -> (First Call?: T/F=w163:bool)
            n72 = case shown="False" w163 {
              tunnel: w171 -> [w180 w198]
              tunnel: [w179 w196] -> w170
              tunnel: w169 -> [w175 w193]
              tunnel: [w178 w197] -> w168
              tunnel: [w177 w195] -> w162
              tunnel: [w176 w194] -> w159
              frame False {
                n73 = Array Size(array=w175) -> (size(s)=w174:i32)
                n74 = for {
                  N: w174 -> [_]
                  shift-right: [w181] -> w179
                  shift-left: w180 -> [w184]
                  tunnel: w175 -> [w187] mode=indexing
                  tunnel: [w182] -> w178 mode=indexing
                  tunnel: [w183] -> w176 mode=indexing
                  tunnel: [w188] -> w177 mode=indexing
                  workers-P: w174 -> [_]
                  n75 = call-dynamic "check_is_moving.vi"("error in (no error)"=w184, "_stage in"=w187) -> ("error out"=w185:errorcluster, "_stage out"=w186:refnum<class "_stage.lvclass">)  [unwired: 7 in, 1 out]
                  n76 = call-dynamic "Read is moving_.vi"("error in (no error)"=w185, "_stage in"=w186) -> ("error out"=w189:errorcluster, "is moving?"=w188:bool, "_stage out"=w190:refnum<class "_stage.lvclass">)  [unwired: 7 in]
                  n77 = call-dynamic "get_curr_position.vi"("error in (no error)"=w189, "_stage in"=w190) -> ("error out"=w181:errorcluster, "readback position"=w191:dbl[], "_stage out"=w182:refnum<class "_stage.lvclass">)  [unwired: 7 in]
                  n78 = Index Array(array=w191) -> (element=w183:dbl)  [unwired: 1 in]
                }
              }
              frame True {
                # "set readback position as first stage position"
                n79 = Array Size(array=w193) -> (size(s)=w192:i32)
                n80 = for {
                  N: w192 -> [_]
                  tunnel: w193 -> [w211] mode=indexing
                  tunnel: [w202] -> w197 mode=indexing
                  tunnel: [w200] -> w195 mode=indexing
                  shift-right: [w201] -> w196
                  shift-left: w198 -> [w210]
                  tunnel: [w199] -> w194 mode=indexing
                  workers-P: w192 -> [_]
                  n81 = call-dynamic "check_is_moving.vi"("error in (no error)"=w210, "_stage in"=w211) -> ("error out"=w208:errorcluster, "Numeric"=w199:dbl, "_stage out"=w209:refnum<class "_stage.lvclass">)  [unwired: 7 in]
                  n82 = Build Array(w199) -> (w207:dbl[])
                  n83 = call-dynamic "Write pos_curr.vi"("error in (no error)"=w208, "set_pos"=w207, "_stage in"=w209) -> ("error out"=w205:errorcluster, "_stage out"=w206:refnum<class "_stage.lvclass">)  [unwired: 7 in]
                  n84 = call-dynamic "check_is_moving.vi"("error in (no error)"=w205, "_stage in"=w206) -> ("error out"=w203:errorcluster, "_stage out"=w204:refnum<class "_stage.lvclass">)  [unwired: 7 in, 1 out]
                  n85 = call-dynamic "Read is moving_.vi"("error in (no error)"=w203, "_stage in"=w204) -> ("error out"=w201:errorcluster, "is moving?"=w200:bool, "_stage out"=w202:refnum<class "_stage.lvclass">)  [unwired: 7 in]
                }
                n86 = local write "stage position(s)"(w194) -> ()
              }
            }
            "stage position(s) readback" <- w159
            n87 = Not(x=w166) -> (.not. x?=w165:bool)
            n88 = property on="trig1 level" class="Slide (strict)"() -> ("Scale.Range"=w158:T12)  [unwired: 2 in, 2 out]
            n89 = property on="Tank 1" class="Slide (strict)"("Scale.Range"=w158) -> ()  [unwired: 2 in, 2 out]
            n90 = Wait (ms)(milliseconds to wait=u32 100) -> ()  [unwired: 1 out]
            n91 = property class="_camera.lvclass"(reference=w160, error in=w161, "stage positions readback"=w159) -> (reference out=w173:refnum<class "_camera.lvclass">, error out=w172:errorcluster)
            n92 = local write "is moving?"(w162) -> ()
          }
          frame Error {
            n93 = Bundle(cluster=w219, "state"=state."stop" ("element")) -> (w217:cluster{"state":T7, "value":variant})  [unwired: 1 in]
            n94 = Enqueue Element(queue=w225, element=w217, error in (no error)=w224) -> ()  [unwired: 1 in, 3 out]
            n95 = Not(x=w213) -> (.not. x?=w212:bool)
            n96 = One Button Dialog(message="timeout caught an error", button name ("OK")="Exit and tell me what's up!") -> ()  [unwired: 1 out]
          }
        }
        "Boolean" <- w145
        n97 = local write "timed out?"(w143) -> ()
        "timed out?" <- w144
      }
      frame "hw_init" {
        n98 = flat-sequence {
          tunnel: w255 -> [w280]
          tunnel: w253 -> [w281]
          tunnel: w252 -> [w279]
          tunnel: [w277] -> w251
          tunnel: [w281] -> w250
          tunnel: [w275] -> w247
          tunnel: w246 -> [w276]
          tunnel: w245 -> [w274]
          tunnel: [w273] -> w244
          tunnel: [w278] -> w241
          tunnel: [w294] -> w249
          tunnel: [w295] -> w254
          tunnel: w251 -> [w295]
          tunnel: w250 -> [w294]
          tunnel: [w290] -> w248
          tunnel: w247 -> [w292]
          tunnel: w244 -> [w291]
          tunnel: [w289] -> w243
          tunnel: [w293] -> w242
          tunnel: w241 -> [w293]
          frame #0 {
            n99 = local read "camera config"() -> (w272:path)
            n100 = for {
              tunnel: w280 -> [w288] mode=indexing
              tunnel: [w283] -> w277 mode=indexing
              shift-right: [w282] -> w278
              shift-left: w279 -> [w287]
              i -> [w284]
              n101 = call-dynamic "set_params.vi"("_stage in"=w288, "error in (no error)"=w287) -> ("_stage out"=w286:refnum<class "_stage.lvclass">, "error out"=w285:errorcluster)  [unwired: 7 in]
              n102 = call-dynamic "Write stage num.vi"("error in (no error)"=w285, "stage num"=w284, "_stage in"=w286) -> ("error out"=w282:errorcluster, "_stage out"=w283:refnum<class "_stage.lvclass">)  [unwired: 7 in]
            }
            n103 = property class="_camera.lvclass"(reference=w276, error in=w274, "config file path"=w272) -> (reference out=w275:refnum<class "_camera.lvclass">, error out=w273:errorcluster)
          }
          frame #1 {
            n104 = call-dynamic "set_params.vi"("error in (no error)"=w291, "_camera in"=w292) -> ("error out"=w289:errorcluster, "_camera out"=w290:refnum<class "_camera.lvclass">)  [unwired: 8 in]
          }
        }
        n105 = Bundle(cluster=w229, "state"=state."dat_send_to_process") -> (w231:cluster{"state":T7, "value":variant})  [unwired: 1 in]
        n106 = Enqueue Element(queue=w227, element=w231, error in (no error)=w228) -> ()  [unwired: 1 in, 3 out]
        n107 = call-dynamic "init_hw.vi"("error in (no error)"=w243, "_camera in"=w248) -> ("error out"=w258:errorcluster, "success ?"=w234:bool, "_camera out"=w260:refnum<class "_camera.lvclass">)  [unwired: 7 in]
        n108 = for {
          tunnel: w254 -> [w271] mode=indexing
          tunnel: [w270] -> w235 mode=indexing
          tunnel: [w269] -> w240 mode=indexing
          shift-right: [w268] -> w239
          shift-left: w242 -> [w267]
          n109 = call-dynamic "init_hw.vi"("error in (no error)"=w267, "_stage in"=w271) -> ("error out"=w268:errorcluster, "Boolean"=w270:bool, "_stage out"=w269:refnum<class "_stage.lvclass">)  [unwired: 7 in]
        }
        "Stage(s) initialized" <- w235
        n110 = Build Array(w234) -> (→"Camera initialised?":bool[])
        n111 = property class="_camera.lvclass"(reference=w260, error in=w258) -> (reference out=w259:refnum<class "_camera.lvclass">, error out=w257:errorcluster, "camera name and version"=→"camera name, version":string)
        n112 = Bundle By Name(cluster=w249, "command"=data_process."init") -> (w232:T6)
        n113 = for {
          tunnel: w240 -> [w266] mode=indexing
          tunnel: [w264] -> w238 mode=indexing
          shift-right: [w263] -> w237
          shift-left: w239 -> [w265]
          tunnel: [w262] -> w236 mode=indexing
          n114 = call-dynamic "Read stage name and version.vi"("error in (no error)"=w265, "_stage in"=w266) -> ("error out"=w263:errorcluster, "stage name and version"=w262:string, "_stage out"=w264:refnum<class "_stage.lvclass">)  [unwired: 7 in]
        }
        n115 = property on="stage name(s)" class="LstBox (strict)"("Item Names"=w236) -> ()  [unwired: 2 in, 2 out]
        "vi running?" <- TRUE
      }
      frame "sw_init" {
        w298 = bool[] [TRUE, TRUE, TRUE, FALSE]
        # "workaround for now"
        n116 = To Variant(anything=w298) -> (Variant=w299:variant)
        n117 = property on="save type" class="Arr (strict)"("Value"=w298) -> ()  [unwired: 2 in, 2 out]
        n118 = Bundle(cluster=w297, "state"=state."dat_update_save_type", "value"=w299) -> (w303:cluster{"state":T7, "value":variant})
        n119 = Enqueue Element(queue=w301, element=w303, error in (no error)=w300) -> ()  [unwired: 1 in, 3 out]
      }
      frame "cam_single_acq" {
        n120 = local read "is moving?"() -> (w312:bool[])
        n121 = Tick Count (ms)() -> (millisecond timer value=w313:u32)
        n122 = Equal To 0?(x="move stage") -> (x = 0?=w315:bool)
        n123 = Or Array Elements(Boolean array=w312) -> (logical OR=w316:bool)
        n124 = And(x=w312, y="indep?") -> (x .and. y?=w310:bool[])
        n125 = And(x=w316, y=w315) -> ()  [unwired: 1 out]
        n126 = Or Array Elements(Boolean array=w310) -> (logical OR=w309:bool)
        n127 = case shown="False" w309 {
          tunnel: w328 -> [w359 w375]
          tunnel: w327 -> [w358 w374]
          tunnel: w326 -> [w357 w370]
          tunnel: [w355 w375] -> w325
          tunnel: [w353 w374] -> w324
          tunnel: w323 -> [w342 w373]
          tunnel: w322 -> [w352 w372]
          tunnel: [w351 w372] -> w321
          tunnel: [w349 w373] -> w320
          tunnel: w319 -> [w345 w383]
          tunnel: w318 -> [w344 w382]
          tunnel: w317 -> [w346 w376]
          tunnel: [w337 w370] -> w314
          tunnel: w313 -> [w330 _]
          frame False {
            n128 = call-dynamic "get_single_acq.vi"("error in (no error)"=w358, "_camera in"=w359) -> ("error out"=w354:errorcluster, "trigger"=w332:dbl[][], "raw data"=w334:i32[][][], "_camera out"=w356:refnum<class "_camera.lvclass">)  [unwired: 6 in]
            n129 = Array Size(array=w342) -> (size(s)=w341:i32)
            n130 = property class="_camera.lvclass"(reference=w356, error in=w354) -> (reference out=w355:refnum<class "_camera.lvclass">, error out=w353:errorcluster, "wavelength"=w335:dbl[])
            n131 = for {
              N: w341 -> [_]
              tunnel: w342 -> [w369] mode=indexing
              tunnel: [w364] -> w350 mode=indexing
              tunnel: [w366] -> w349 mode=indexing
              shift-right: [w367] -> w351
              shift-left: w352 -> [w368]
              workers-P: w341 -> [_]
              n132 = call-dynamic "get_curr_position.vi"("error in (no error)"=w368, "_stage in"=w369) -> ("error out"=w367:errorcluster, "readback position"=w365:dbl[], "_stage out"=w366:refnum<class "_stage.lvclass">)  [unwired: 7 in]
              n133 = Index Array(array=w365) -> (element=w364:dbl)  [unwired: 1 in]
            }
            n134 = Build Array("trig1 level", "trig2 level") -> (w339:dbl[])
            n135 = for {
              tunnel: w332 -> [w363] mode=indexing
              tunnel: [w362] -> w333 mode=indexing
              tunnel: w339 -> [w361] mode=indexing
              n136 = Greater?(x=w363, y=w361) -> (0:w362:bool[])
            }
            n137 = Bundle(cluster=w346, "state"=state."dat_send_to_process") -> (w348:cluster{"state":T7, "value":variant})  [unwired: 1 in]
            n138 = Enqueue Element At Opposite End(queue=w344, element=w348, error in (no error)=w345) -> ()  [unwired: 1 in, 3 out]
            n139 = local write "stage position(s) readback"(w350) -> ()
            n140 = Bundle By Name(cluster=w357, "command"=data_process."process", "wavelength"=w335, "raw data"=w334, "trigger"=w333, "raw PDs"=w332) -> (w337:T6)
            n141 = local read "millisecond timer value"() -> (w329:u32)
            "cont acq. time" <- w329
            n142 = flat-sequence {
              tunnel: w337 -> [_]
              tunnel: [w360] -> w331
              frame #0 {
                n143 = Tick Count (ms)() -> (millisecond timer value=w360:u32)
              }
            }
            n144 = Subtract(x=w331, y=w330) -> (x-y=→"single acq. time":u32)
            n145 = Subtract(x=w329, y=w330) -> ()  [unwired: 1 out]
            "millisecond timer value 2" <- w330
          }
          frame True {
            # "need to reverse order when enqueuing at opposite end !!!!!!"
            n146 = Bundle(cluster=w376, "state"=state."cam_single_acq") -> (w381:cluster{"state":T7, "value":variant})  [unwired: 1 in]
            n147 = Enqueue Element At Opposite End(queue=w382, element=w381, error in (no error)=w383) -> (queue out=w378:refnum<queue>, error out=w377:errorcluster)  [unwired: 1 in, 1 out]
            n148 = Bundle(cluster=w376, "state"=state."timeout") -> (w379:cluster{"state":T7, "value":variant})  [unwired: 1 in]
            n149 = Enqueue Element At Opposite End(queue=w378, element=w379, error in (no error)=w377) -> ()  [unwired: 1 in, 3 out]
          }
        }
      }
      frame "cam_get_bg" {
        n150 = call-dynamic "get_single_acq.vi"("error in (no error)"=w390, "_camera in"=w395) -> ("error out"=w389:errorcluster, "raw data"=w392:i32[][][], "_camera out"=w394:refnum<class "_camera.lvclass">)  [unwired: 6 in, 1 out]
        n151 = for {
          tunnel: [w399] -> w391 mode=indexing
          tunnel: w392 -> [w397] mode=indexing
          n152 = Transpose 2D Array(2D array=w397) -> (transposed array=w398:i32[][])
          n153 = for {
            tunnel: w398 -> [w401] mode=indexing
            tunnel: [w400] -> w399 mode=indexing
            n154 = call-poly <vilib>:"Mean.vi"("X"=w401) -> ("mean"=w400:dbl)  [unwired: 1 out]
          }
        }
        n155 = property class="_camera.lvclass"(reference=w394, error in=w389, "background"=w391) -> (reference out=w393:refnum<class "_camera.lvclass">, error out=w384:errorcluster)
        n156 = flat-sequence {
          tunnel: w384 -> [_]
          frame #0 {
            n157 = local write "Boolean 3"(FALSE ("Boolean 3")) -> ()
          }
        }
        "Boolean 3" <- TRUE
      }
      frame "cam_rst_bg" {
        n158 = property class="_camera.lvclass"(reference=w409, error in=w406, "background"=i32[][] []) -> (reference out=w408:refnum<class "_camera.lvclass">, error out=w405:errorcluster)
      }
      frame "cam_cnt_acq" {
        # "need to make sure that safe flag is false"
        n159 = Tick Count (ms)() -> (millisecond timer value=→"millisecond timer value":u32)
        n160 = Bundle(cluster=w415, "state"=state."cam_single_acq") -> (w421:cluster{"state":T7, "value":variant})  [unwired: 1 in]
        n161 = Enqueue Element(queue=w429, element=w421, error in (no error)=w428) -> (queue out=w427:refnum<queue>, error out=w426:errorcluster)  [unwired: 1 in, 1 out]
        n162 = Bundle(cluster=w415, "state"=state."timeout" ("element")) -> (w419:cluster{"state":T7, "value":variant})  [unwired: 1 in]
        n163 = Enqueue Element(queue=w427, element=w419, error in (no error)=w426) -> (queue out=w416:refnum<queue>, error out=w417:errorcluster)  [unwired: 1 in, 1 out]
        n164 = property on="history length" class="DigNum (strict)"("Value"=30 ("history length")) -> ()  [unwired: 2 in, 2 out]
        n165 = Bundle(cluster=w415, "state"=state."cam_cnt_acq") -> (w418:cluster{"state":T7, "value":variant})  [unwired: 1 in]
        n166 = Enqueue Element(queue=w416, element=w418, error in (no error)=w417) -> ()  [unwired: 1 in, 3 out]
      }
      frame "cam_set_wl" {
        # "Hartmann dispersion formula:\nd(\\lambda) = a1 + a2 / (pix - a3)"
        n167 = Variant To Data(type=TRUE, Variant=w446) -> (data=w445:bool)  [unwired: 1 in, 1 out]
        n168 = property class="_camera.lvclass"(reference=w453, error in=w452) -> (reference out=w451:refnum<class "_camera.lvclass">, "wavelength"=w432:dbl[])  [unwired: 1 out]
        n169 = Array Size(array=w432) -> (size(s)=w431:i32)
        n170 = for {
          N: w431 -> [_]
          tunnel: [w459] -> w430 mode=indexing
          i -> [w459]
        }
        n171 = case shown="True" w445 {
          tunnel: [w463 w476] -> w440
          tunnel: [w463 w464] -> w436
          tunnel: [w463 w479] -> w439
          tunnel: [w463 w475] -> w447
          tunnel: "pixel/index" -> [_ w467]
          tunnel: "wavelength \n(calibration value)" -> [_ w466]
          tunnel: T11 {"model"="a1+a2/(x-a3)", "Parameters"=["a1", "a2", "a3"], "x"="x"} ("model description") -> [_ w465]
          tunnel: w430 -> [w463 w464]
          frame False {
          }
          frame True {
            n172 = Sort 1D Array(array=w466) -> (sorted array=w478:dbl[])
            n173 = Sort 1D Array(array=w467) -> (sorted array=w476:u16[])
            n174 = case shown="True" "mirror?" {
              tunnel: w478 -> [w480 w482]
              tunnel: [w480 w481] -> w475
              frame False {
              }
              frame True {
                n175 = Reverse 1D Array(array=w482) -> (reversed array=w481:dbl[])
              }
            }
            n176 = call-poly <vilib>:"Nonlinear Curve Fit.vi"("Y"=w475, "initial parameters"="initial parameters", "X"=w476, "model description"=w465) -> ("best fit parameters"=w473:dbl[])  [unwired: 7 in, 4 out]
            "best fit parameters" <- w473
            n177 = Index Array(array=w473) -> (element #1=w472:dbl, element #2=w471:dbl, element #3=w469:dbl)  [unwired: 3 in]
            n178 = Subtract(x=w464, y=w469) -> (x-y=w470:dbl[])
            n179 = Divide(x=w471, y=w470) -> (x/y=w468:dbl[])
            n180 = Add(x=w472, y=w468) -> (x+y=w479:dbl[])
          }
        }
        n181 = for {
          tunnel: "pixel/index" -> [w462] mode=indexing
          tunnel: w439 -> [w461]
          tunnel: [w460] -> w443 mode=indexing
          n182 = Index Array(array=w461, index=w462) -> (element=w460:dbl)
        }
        "wavelength (fitted)" <- w443
        n183 = Subtract(x="wavelength \n(calibration value)", y=w443) -> (x-y=w442:dbl[])
        n184 = Subtract(x=w439, y=w439) -> (x-y=w438:dbl[])
        n185 = property class="_camera.lvclass"(reference=w451, "wavelength"=w439) -> (reference out=w458:refnum<class "_camera.lvclass">, error out=w457:errorcluster)  [unwired: 1 in]
        n186 = Bundle(w440, w447) -> (w450:cluster{i32[], dbl[]})  [unwired: 1 in]
        n187 = Bundle(w436, w439) -> (w449:cluster{i32[], dbl[]})  [unwired: 1 in]
        n188 = Bundle("pixel/index"="pixel/index", w442) -> (w441:cluster{"pixel/index":u16[], dbl[]})  [unwired: 1 in]
        n189 = Bundle(w436, w438) -> (w437:cluster{i32[], dbl[]})  [unwired: 1 in]
        n190 = Build Array(w450, w449, w441, w437) -> (→"wavelength fit":cluster{"pixel/index":i32[], dbl[]}[])
      }
      frame "stg_set_pos" {
        # "parallel execution of for loop\nto address stages more or less\nsimultaneously"
        # "parallel execution of for loop"
        # "find out which stage was moved"
        n191 = property class="_camera.lvclass"(reference=w497) -> (reference out=w496:refnum<class "_camera.lvclass">, "stage positions"=w495:dbl[])  [unwired: 1 in, 1 out]
        n192 = Array Size(array=w485) -> (size(s)=w484:i32)
        n193 = Variant To Data(type=dbl[] [], Variant=w500) -> (data=w492:dbl[])  [unwired: 1 in, 1 out]
        n194 = for {
          N: w484 -> [_]
          tunnel: w485 -> [w509] mode=indexing
          tunnel: [w505] -> w490 mode=indexing
          shift-right: [w504] -> w489
          shift-left: w491 -> [w508]
          tunnel: [w503] -> w488 mode=indexing
          workers-P: w484 -> [_]
          n195 = call-dynamic "check_is_moving.vi"("error in (no error)"=w508, "_stage in"=w509) -> ("error out"=w506:errorcluster, "_stage out"=w507:refnum<class "_stage.lvclass">)  [unwired: 7 in, 1 out]
          n196 = call-dynamic "Read is moving_.vi"("error in (no error)"=w506, "_stage in"=w507) -> ("error out"=w504:errorcluster, "is moving?"=w503:bool, "_stage out"=w505:refnum<class "_stage.lvclass">)  [unwired: 7 in]
        }
        n197 = for {
          tunnel: w492 -> [w531] mode=indexing
          tunnel: w495 -> [w529]
          tunnel: [w530] -> w487 mode=indexing
          i -> [w528]
          n198 = Index Array(array=w529, index=w528) -> (element=w527:dbl)
          n199 = Not Equal?(x=w531, y=w527) -> (x != y?=w530:bool)
        }
        n200 = Or(x=w487, y=w488) -> (x .or. y?=w486:bool[])
        "is moving?" <- w486
        n201 = property on="stage position(s)" class="Arr (strict)"("Value"=w492) -> ()  [unwired: 2 in, 2 out]
        n202 = property class="_camera.lvclass"(reference=w496, "stage positions"=w492) -> (reference out=w501:refnum<class "_camera.lvclass">)  [unwired: 1 in, 1 out]
        n203 = Array Size(array=w490) -> (size(s)=w483:i32)
        n204 = for {
          N: w483 -> [_]
          tunnel: w490 -> [w518] mode=indexing
          tunnel: w486 -> [w512]
          tunnel: [w517] -> w494 mode=indexing
          shift-right: [w516] -> w493
          shift-left: w489 -> [w515]
          tunnel: w492 -> [w514]
          workers-P: w483 -> [_]
          i -> [w511]
          n205 = Index Array(array=w514, index=w511) -> (element=w513:dbl)
          n206 = Index Array(array=w512, index=w511) -> (element=w510:bool)
          n207 = case shown="True" w510 {
            tunnel: w518 -> [w520 w526]
            tunnel: [w520 w524] -> w517
            tunnel: [w519 w522] -> w516
            tunnel: w515 -> [w519 w523]
            tunnel: w513 -> [_ w521]
            frame False {
            }
            frame True {
              n208 = Build Array(w521) -> (w525:dbl[])
              n209 = call-dynamic "set_new_position.vi"("error in (no error)"=w523, "set_pos"=w525, "_stage in"=w526) -> ("error out"=w522:errorcluster, "_stage out"=w524:refnum<class "_stage.lvclass">)  [unwired: 7 in]
            }
          }
        }
        "Stage objects" <- w494
      }
      frame "stg_home" {
      }
      frame "scn_load_step_file" {
        n210 = Variant To Data(type=path "", Variant=w559) -> (data=w557:path)  [unwired: 1 in, 1 out]
        n211 = call-poly <vilib>:"Read Delimited Spreadsheet.vi"("file path (dialog if empty)"=w557, "transpose? (F)"=TRUE) -> ("all rows"=w537:dbl[][])  [unwired: 8 in, 5 out]
        n212 = Bundle By Name(cluster=w555, "scn_step_time_dly (set) [fs]"=w537) -> (w554:T6)
        n213 = Transpose 2D Array(2D array=w537) -> (transposed array=w540:dbl[][])
        "timesteps loaded from file" <- w540
        n214 = Array Size(array=w540) -> (size(s)=w543:i32[])
        n215 = Index Array(array=w540, index (col)=0 ("index (row)")) -> (element=w539:dbl[])  [unwired: 1 in]
        n216 = Index Array(array=w543, index=1) -> (element=w542:i32)
        n217 = case shown="1" w542 {
          tunnel: w539 -> [_ w563]
          frame 0, Default {
          }
          frame 1 {
            "Waveform Graph" <- w563
          }
        }
        n218 = Array Size(array=w537) -> (size(s)=w550:i32[])
        n219 = Array Size(array=w548) -> (size(s)=w546:i32)
        n220 = Index Array(array=w550) -> (element=w547:i32)  [unwired: 1 in]
        n221 = Decrement(x=w547) -> (x-1=w549:i32)
        n222 = Greater?(x=w547, y=w546) -> (0:w545:bool)
        n223 = Index Array(array=w537, index (row)=w549) -> (element=w553:dbl[])  [unwired: 1 in]
        n224 = for {
          tunnel: w537 -> [w566] mode=indexing
          tunnel: [w564] -> w544 mode=indexing
          n225 = call "Remove Duplicates From 1D Array.vim"("array"=w566) -> ("array with duplicates removed"=w565:dbl[])  [unwired: 10 in]
          n226 = Array Size(array=w565) -> (size(s)=w564:i32)
        }
        "Array" <- w544
        n227 = call "Remove Duplicates From 1D Array.vim"("array"=w553) -> ("array with duplicates removed"=w552:dbl[])  [unwired: 10 in]
        n228 = case shown="True" w545 {
          frame False {
          }
          frame True {
            n229 = One Button Dialog(message="Be careful, timestep file dimension exceeds number of stages.", button name ("OK")="\"I like to live dangerously!\"") -> ()  [unwired: 1 out]
          }
        }
        n230 = Array Size(array=w552) -> (size(s)=→"size of dependent time scan":i32)
      }
      frame "scn_init" {
        w570 = 0 ("scn_iter")
        n231 = Unbundle By Name(w583) -> ("scn_step_time_dly (set) [fs]"=w576:dbl[][])
        n232 = property on="cont acq" class="Bool (strict)"("Value"=FALSE ("cont acq")) -> ()  [unwired: 2 in, 2 out]
        n233 = for {
          tunnel: w576 -> [w594] mode=indexing
          tunnel: [w592] -> w575 mode=indexing
          n234 = call "Remove Duplicates From 1D Array.vim"("array"=w594) -> ("array with duplicates removed"=w593:dbl[])  [unwired: 10 in]
          n235 = Array Size(array=w593) -> (size(s)=w592:i32)
        }
        n236 = Index Array(array=w575) -> (element=w574:i32)  [unwired: 1 in]
        n237 = Empty Array?(array=w576) -> (empty?=w587:bool)
        n238 = case shown="False" w587 {
          tunnel: w586 -> [w600 w609]
          tunnel: w585 -> [w599 w608]
          tunnel: w584 -> [w598 w603]
          tunnel: w574 -> [w597 _]
          frame False {
            n239 = Add(x=w597, y=10) -> (x+y=w596:i32)
            n240 = property on="history length" class="DigNum (strict)"("Value"=w596) -> ()  [unwired: 2 in, 2 out]
            n241 = Bundle(cluster=w598, "state"=state."scn_next_step") -> (w602:cluster{"state":T7, "value":variant})  [unwired: 1 in]
            n242 = Enqueue Element(queue=w600, element=w602, error in (no error)=w599) -> ()  [unwired: 1 in, 3 out]
          }
          frame True {
            n243 = Bundle(cluster=w603, "state"=state."scn_load_step_file") -> (w611:cluster{"state":T7, "value":variant})  [unwired: 1 in]
            n244 = Enqueue Element(queue=w609, element=w611, error in (no error)=w608) -> (queue out=w605:refnum<queue>, error out=w604:errorcluster)  [unwired: 1 in, 1 out]
            n245 = Bundle(cluster=w603, "state"=state."scn_init") -> (w607:cluster{"state":T7, "value":variant})  [unwired: 1 in]
            n246 = Enqueue Element(queue=w605, element=w607, error in (no error)=w604) -> ()  [unwired: 1 in, 3 out]
          }
        }
        n247 = local read "N scans"() -> (w580:u16)
        n248 = call "create_save_dir_and_fn.vi"("scn_iter"=w570, "sample"="sample", "Experiment"="Experiment", "data folder"="data folder") -> ("Path"=w571:path)  [unwired: 7 in]
        n249 = property on="progress" class="Slide (strict)"("Scale.Maximum"=w580, "Scale.Minimum"=0.0 ("Scale.Range:Minimum")) -> ()  [unwired: 2 in, 2 out]
        n250 = Bundle By Name(cluster=w583, "scn_step"=-1, "save path"=w571, "scn_iter"=w570, "scan done?"=FALSE) -> (w581:T6)
        n251 = local write "current scan"(w570) -> ()
      }
      frame "scn_next_step" {
        n252 = Unbundle By Name(w628) -> ("scn_step_time_dly (set) [fs]"=w622:dbl[][], "scn_step"=w617:i32, "scn_iter"=w625:i32)
        n253 = Index Array(array=w622) -> (element=w623:dbl[])  [unwired: 2 in]
        n254 = local read "t0 position(s)"() -> (w624:dbl[])
        n255 = Array Size(array=w623) -> (size(s)=w618:i32)
        n256 = Increment(x=w617) -> (x+1=w613:i32)
        "scan progress" <- w613
        n257 = Add(x=w625, y=0.5) -> (x+y=→"progress":dbl)
        n258 = Increment(x=w625) -> (x+1=→"current scan":i32)
        n259 = Greater?(x=w618, y=w613) -> (0:w627:bool)
        n260 = property on="scan progress" class="Slide (strict)"("Scale.Maximum"=w618, "Scale.Minimum"=0.0 ("Scale.Range:Minimum")) -> ()  [unwired: 2 in, 2 out]
        n261 = case shown="False" w627 {
          tunnel: w631 -> [w647 w679]
          tunnel: w630 -> [w646 w678]
          tunnel: w629 -> [w645 w664]
          tunnel: w628 -> [w643 w662]
          tunnel: [w643 w661] -> w615
          tunnel: w622 -> [_ w658]
          tunnel: w613 -> [_ w649]
          tunnel: w624 -> [_ w659]
          tunnel: [w642 w649] -> _
          tunnel: w617 -> [w642 _]
          frame False {
            n262 = Bundle(cluster=w645, "state"=state."scn_next_iter") -> (w648:cluster{"state":T7, "value":variant})  [unwired: 1 in]
            n263 = Enqueue Element(queue=w647, element=w648, error in (no error)=w646) -> ()  [unwired: 1 in, 3 out]
          }
          frame True {
            n264 = Boolean To (0,1)(Boolean="reversed?") -> (0, 1=w655:i16[])
            n265 = Multiply(x=w655, y=2) -> (x*y=w653:i32[])
            n266 = Index Array(array=w658, index (col)=w649) -> (element=w650:dbl[])  [unwired: 1 in]
            n267 = Subtract(x=w653, y=1) -> (x-y=w651:i32[])
            n268 = Multiply(x=w651, y=w650) -> (x*y=w657:dbl[])
            n269 = Subtract(x=w659, y=w657) -> (x-y=w660:dbl[])
            n270 = Bundle(cluster=w664, "state"=state."stg_set_pos", "value"=w660) -> (w677:cluster{"state":T7, "value":variant})
            n271 = Enqueue Element(queue=w679, element=w677, error in (no error)=w678) -> (queue out=w674:refnum<queue>, error out=w673:errorcluster)  [unwired: 1 in, 1 out]
            n272 = Bundle By Name(cluster=w662, "scn_step"=w649) -> (w661:T6)
            n273 = Bundle(cluster=w664, "state"=state."cam_single_acq") -> (w675:cluster{"state":T7, "value":variant})  [unwired: 1 in]
            n274 = Enqueue Element(queue=w674, element=w675, error in (no error)=w673) -> (queue out=w670:refnum<queue>, error out=w669:errorcluster)  [unwired: 1 in, 1 out]
            n275 = Bundle(cluster=w664, "state"=state."timeout") -> (w671:cluster{"state":T7, "value":variant})  [unwired: 1 in]
            n276 = Enqueue Element(queue=w670, element=w671, error in (no error)=w669) -> (queue out=w666:refnum<queue>, error out=w665:errorcluster)  [unwired: 1 in, 1 out]
            n277 = Bundle(cluster=w664, "state"=state."scn_next_step") -> (w667:cluster{"state":T7, "value":variant})  [unwired: 1 in]
            n278 = Enqueue Element(queue=w666, element=w667, error in (no error)=w665) -> ()  [unwired: 1 in, 3 out]
          }
        }
        n279 = Increment(x=w613) -> (x+1=w612:i32)
        n280 = Greater?(x=w618, y=w612) -> (0:w616:bool)
        n281 = case shown="True" w616 {
          tunnel: w615 -> [w638 w640]
          tunnel: [w637 w639] -> w614
          frame False {
            n282 = Bundle By Name(cluster=w638, "scan done?"=TRUE) -> (w637:T6)
          }
          frame True {
            n283 = Bundle By Name(cluster=w640, "scan done?"=FALSE) -> (w639:T6)
          }
        }
      }
      frame "scn_next_iter" {
        n284 = Unbundle By Name(w686) -> ("save path"=w685:path, "scn_iter"=w684:i32)
        n285 = Unbundle By Name(w686) -> ("scn_iter"=w683:i32)
        n286 = Decrement(x="N scans") -> (x-1=w682:u16)
        n287 = Less?(x=w683, y=w682) -> (x < y?=w694:bool)
        n288 = case shown="True" w694 {
          tunnel: w686 -> [w695 w721]
          tunnel: w693 -> [w700 w717]
          tunnel: w692 -> [w699 w716]
          tunnel: w691 -> [_ w715]
          tunnel: w685 -> [_ w714]
          tunnel: w684 -> [w697 w704]
          tunnel: [w695 w701] -> w680
          frame False {
            n289 = Increment(x=w697) -> (x+1=w696:i32)
            n290 = Flush Queue(queue=w700, error in (no error)=w699) -> ()  [unwired: 3 out]
            n291 = local write "progress"(w696) -> ()
            n292 = property on="scan" class="Bool (strict)"("Value"=FALSE ("scan")) -> ()  [unwired: 2 in, 2 out]
          }
          frame True {
            n293 = Strip Path(path=w714) -> (stripped path=w705:path, name=w709:string)
            n294 = Increment(x=w704) -> (x+1=w703:i32)
            n295 = String Length(string=w709) -> (length=w713:i32)
            n296 = Bundle(cluster=w715, "state"=state."scn_next_step") -> (w719:cluster{"state":T7, "value":variant})  [unwired: 1 in]
            n297 = Subtract(x=w713, y=3) -> (x-y=w711:i32)
            n298 = String Subset(string=w709, length (rest)=w711) -> (substring=w710:string)  [unwired: 1 in]
            n299 = Enqueue Element(queue=w717, element=w719, error in (no error)=w716) -> ()  [unwired: 1 in, 3 out]
            n300 = Format Into String(format string="%03d", w703) -> (resulting string=w707:string)  [unwired: 2 in, 1 out]
            n301 = Concatenate Strings(w710, w707) -> (w706:string)
            n302 = Build Path(base path=w705, name or relative path=w706) -> (appended path=w702:path)
            n303 = Bundle By Name(cluster=w721, "scn_step"=-1, "save path"=w702, "scn_iter"=w703) -> (w701:T6)
          }
        }
      }
      frame "dat_update_save_flag" {
        n304 = Variant To Data(type=FALSE, Variant=w724) -> (data=w722:bool)  [unwired: 1 in, 1 out]
        n305 = Bundle By Name(cluster=w730, "save flag"=w722) -> (w729:T6)
      }
      frame "dat_update_save_type" {
        n306 = Variant To Data(type=bool[] [], Variant=w735) -> (data=w731:bool[])  [unwired: 1 in, 1 out]
        n307 = Bundle By Name(cluster=w737, "save type"=w731) -> (w736:T6)
      }
      frame "dat_save_raw" {
        n308 = To Variant(anything=bool[] [FALSE, FALSE, FALSE, TRUE]) -> (Variant=w767:variant)
        n309 = Bundle(cluster=w759, "state"=state."dat_update_save_type", "value"=w767) -> (w770:cluster{"state":T7, "value":variant})
        n310 = local read "data folder"() -> (w743:path)
        n311 = Enqueue Element(queue=w769, element=w770, error in (no error)=w768) -> (queue out=w763:refnum<queue>, error out=w762:errorcluster)  [unwired: 1 in, 1 out]
        n312 = Get Date/Time In Seconds() -> (seconds since 1Jan1904=w746:timestamp)
        n313 = Format Date/Time String(time format string (%c)="%Y%m%d", seconds (now)=w746) -> (date/time string=w748:string)  [unwired: 1 in]
        n314 = Build Path(base path=w743, name or relative path=w748) -> (appended path=w745:path)
        n315 = Bundle(cluster=w759, "state"=state."cam_single_acq") -> (w764:cluster{"state":T7, "value":variant})  [unwired: 1 in]
        n316 = Enqueue Element(queue=w763, element=w764, error in (no error)=w762) -> (queue out=w758:refnum<queue>, error out=w757:errorcluster)  [unwired: 1 in, 1 out]
        n317 = Build Path(base path=w745, name or relative path="raw_acquisition") -> (appended path=w742:path)
        n318 = Build Path(base path=w742, name or relative path="raw") -> (appended path=w740:path)
        n319 = Unbundle By Name(w750) -> ("save type"=w754:bool[])
        n320 = Bundle By Name(cluster=w750, "save path"=w740) -> (w749:T6)
        n321 = To Variant(anything=w754) -> (Variant=w753:variant)
        n322 = Bundle(cluster=w759, "state"=state."dat_update_save_type", "value"=w753) -> (w760:cluster{"state":T7, "value":variant})
        n323 = Enqueue Element(queue=w758, element=w760, error in (no error)=w757) -> ()  [unwired: 1 in, 3 out]
      }
      frame "dat_send_to_process" {
        n324 = Variant To Data(type=TRUE, Variant=w778) -> (data=w776:bool, error out=w775:errorcluster)  [unwired: 1 in]
        n325 = case shown="No Error" w775 {
          tunnel: w776 -> [w783 _]
          frame No Error {
            n326 = case shown="False" w783 {
              frame False {
              }
              frame True {
              }
            }
          }
          frame Error {
          }
        }
        n327 = Enqueue Element(queue=w774, element=w772, error in (no error)=w773) -> ()  [unwired: 1 in, 3 out]
      }
      frame "aux_save_wl_to_ini" {
        n328 = call <vilib>:"Application Directory.vi"() -> ("Application Directory"=w790:path)
        n329 = local read "wavelength \n(calibration value)"() -> (w787:dbl[])
        n330 = Build Path(base path=w790, name or relative path="cameras\\spectral_calibration.ini") -> (appended path=w785:path)
        n331 = local read "best fit parameters"() -> (w788:dbl[])
        n332 = local read "pixel/index"() -> (w784:u16[])
        n333 = call "save_wl_to_config.vi"("wavelength \n(calibration value)"=w787, "best fit parameters"=w788, "appended path"=w785, "pix"=w784) -> ("error out"=w786:errorcluster)  [unwired: 7 in]
        n334 = call <vilib>:"Simple Error Handler.vi"("error in (no error)"=w786) -> ()  [unwired: 4 in, 5 out]
      }
      frame "aux_center_cursor" {
        n335 = property on="main graph" class="XYGraph (strict)"() -> ("CrsrList"=w796:T13)  [unwired: 2 in, 2 out]
        n336 = for {
          tunnel: w796 -> [_] mode=indexing
          i -> [w802]
          n337 = property on="main graph" class="XYGraph (strict)"("Active Cursor"=w802, "Cursor.Cursor X"=500.0 ("Cursor.Cursor Position:Cursor X")) -> ()  [unwired: 2 in, 2 out]
        }
      }
      frame "stop" {
        w828 = TRUE
        n338 = for {
          tunnel: w821 -> [w833] mode=indexing
          tunnel: [w830] -> w818 mode=indexing
          shift-right: [w831] -> w819
          shift-left: w820 -> [w832]
          n339 = call-dynamic "close_hw.vi"("error in (no error)"=w832, "_stage in"=w833) -> ("error out"=w831:errorcluster, "_stage out"=w830:refnum<class "_stage.lvclass">)  [unwired: 8 in]
        }
        n340 = Bundle(cluster=w809, "state"=state."dat_send_to_process", "value"=TRUE) -> (w811:cluster{"state":T7, "value":variant})
        n341 = Enqueue Element(queue=w815, element=w811, error in (no error)=w814) -> (queue out=w812:refnum<queue>, error out=w813:errorcluster)  [unwired: 1 in, 1 out]
        n342 = call-dynamic "release_hw.vi"("error in (no error)"=w824, "_camera in"=w827) -> ("error out"=w822:errorcluster, "_camera out"=w826:refnum<class "_camera.lvclass">)  [unwired: 8 in]
        n343 = Release Queue(queue=w812, error in (no error)=w813) -> ()  [unwired: 1 in, 3 out]
        n344 = Bundle By Name(cluster=w823, "command"=data_process."exit") -> (w805:T6)
        n345 = Build Array(FALSE ("camera initialized?")) -> (w816:bool[])
        n346 = Enqueue Element(queue=w807, element=w805, error in (no error)=w806) -> ()  [unwired: 1 in, 3 out]
        n347 = local write "Stage(s) initialized"(bool[] [FALSE] ("Stage(s) initialized")) -> ()
        n348 = local write "Camera initialised?"(w816) -> ()
        n349 = Not(x=w828) -> (.not. x?=w829:bool)
        n350 = local write "vi running?"(w829) -> ()
      }
    }
    n351 = Merge Errors(w132, w130) -> (w131:errorcluster)
  }
  n352 = while {
    border: w89 -> [_]
    shift-right: [w834] -> _
    shift-left: w74 -> [w835]
    tunnel: w69 -> [w842]
    stop <- w845 stop-if-true
    # "handle timeout\ncases here"
    # "Data processing and visualisation"
    n353 = Dequeue Element(queue=w842, timeout in ms (-1)=5) -> (queue out=w839:refnum<queue>, element=w838:T6, timed out?=w840:bool, error out=w837:errorcluster)  [unwired: 1 in]
    n354 = Unbundle By Name(w838) -> ("command"=w836:T5)
    n355 = Select(t=data_process."timeout", s=w840, f=w836) -> (s? t:f=w843:T5)
    n356 = case shown="\"plot\"" w843 {
      tunnel: [_ _ _ _ _ _ _ TRUE] -> w845
      tunnel: w835 -> [w869 w886 w892 w939 w1004 w1150 w1152 w1206]
      tunnel: [w869 w884 w890 w904 w1004 w1150 w1152 w1206] -> w834
      tunnel: w839 -> [_ _ _ w937 w1012 _ _ w1205]
      tunnel: w838 -> [_ _ _ w908 w1009 w1148 w1153 _]
      tunnel: w837 -> [_ _ _ w936 w1011 _ _ _]
      frame "timeout", Default {
        w848 = 100.0
        n357 = local read "PDs std"() -> (w860:dbl[])
        n358 = local read "PDs mean"() -> (w861:dbl[])
        n359 = property on="skipped" class="Arr (strict)"() -> ("Value"=w865:bool[])  [unwired: 2 in, 2 out]
        n360 = Multiply(x=w860, y=5.0) -> (x*y=w859:dbl[])
        n361 = Index Array(array=w865) -> (element=→"Boolean 2":bool)  [unwired: 1 in]
        n362 = Add(x=w861, y=w859) -> (x+y=w854:dbl[])
        n363 = Subtract(x=w861, y=w859) -> (x-y=w853:dbl[])
        n364 = Divide(x=w854, y=w848) -> (x/y=w852:dbl[])
        n365 = Divide(x=w853, y=w848) -> (x/y=w851:dbl[])
        n366 = Round Toward +Infinity(x=w852) -> (ceil(x): smallest int >= x=w850:dbl[])
        n367 = Round Toward -Infinity(1:w851) -> (0:w849:dbl[])
        n368 = Multiply(x=w850, y=w848) -> (x*y=w847:dbl[])
        n369 = Multiply(x=w849, y=w848) -> (x*y=w846:dbl[])
        n370 = control-ref of="PD"() -> (w857:refnum<vi>)
        n371 = control-ref of="PD hist"() -> (w856:refnum<vi>)
        n372 = Build Array(w857, w856) -> (w855:refnum<vi>[])
        n373 = property on="trig1 level" class="Slide (strict)"() -> ("Scale.Range"=w863:T12)  [unwired: 2 in, 2 out]
        n374 = property on="trig2 level" class="Slide (strict)"() -> ("Scale.Range"=w862:T12)  [unwired: 2 in, 2 out]
        n375 = property on="main graph" class="XYGraph (strict)"() -> ("CrsrList"=w866:T13)  [unwired: 2 in, 2 out]
        n376 = for {
          tunnel: w855 -> [w874] mode=indexing
          tunnel: w847 -> [w873]
          tunnel: w846 -> [w871]
          n377 = Index Array(array=w873) -> (element=w872:dbl)  [unwired: 1 in]
          n378 = Index Array(array=w871) -> (element=w870:dbl)  [unwired: 1 in]
          n379 = property on="Property Node" class="XYGraph (strict)"(reference=w874, "YScale.Maximum"=w872, "YScale.Minimum"=w870) -> ()  [unwired: 1 in, 2 out]
        }
        n380 = for {
          tunnel: [w877] -> w867 mode=indexing
          tunnel: w866 -> [w876] mode=indexing
          n381 = Bundle By Name(cluster=w876, "Plot"="which plot") -> (w877:T14)
        }
        n382 = property on="Tank 1" class="Slide (strict)"("Scale.Range"=w863) -> ()  [unwired: 2 in, 2 out]
        n383 = property on="Tank 1 + std" class="Slide (strict)"("Scale.Range"=w863) -> ()  [unwired: 2 in, 2 out]
        n384 = property on="Tank 1 - std" class="Slide (strict)"("Scale.Range"=w863) -> ()  [unwired: 2 in, 2 out]
        n385 = property on="Tank 2" class="Slide (strict)"("Scale.Range"=w862) -> ()  [unwired: 2 in, 2 out]
        n386 = property on="Tank 2 - std" class="Slide (strict)"("Scale.Range"=w862) -> ()  [unwired: 2 in, 2 out]
        n387 = property on="Tank 2 + std" class="Slide (strict)"("Scale.Range"=w862) -> ()  [unwired: 2 in, 2 out]
        n388 = property on="main graph" class="XYGraph (strict)"("CrsrList"=w867) -> ()  [unwired: 2 in, 2 out]
        "Tab Control" <- "bottom panel"
      }
      frame "init" {
        w878 = dbl[] []
        w887 = cluster{dbl, u32}[] [{-10000.0, 1187327}, {-5000.0, 7471035}, {0.0, 16448250}, {5000.0, 16773000}, {10000.0, 16747656}] ("Z Scale.Marker Values[]")
        # "init all graphs here"
        n389 = Bundle(w878, w878) -> (w883:cluster{dbl[], dbl[]})  [unwired: 1 in]
        n390 = Bundle(w878, w878) -> (w882:cluster{dbl[], dbl[]})  [unwired: 1 in]
        n391 = Bundle(w878, w878) -> (w881:cluster{dbl[], dbl[]})  [unwired: 1 in]
        n392 = Bundle(w878, w878) -> (w880:cluster{dbl[], dbl[]})  [unwired: 1 in]
        n393 = Build Array(w883, w882, w881, w880) -> (→"main graph":cluster{dbl[], dbl[]}[])
        n394 = property on="Intensity Chart" class="IntChart (strict)"("ZScale.MarkerVals[]"=w887) -> ()  [unwired: 2 in, 2 out]
        n395 = property on="Intensity Graph" class="IntGraph (strict)"("ZScale.MarkerVals[]"=w887) -> ()  [unwired: 2 in, 2 out]
        n396 = Bundle By Name(cluster=w886, "curr acq"=0) -> (w884:T8)
      }
      frame "reset" {
        n397 = Initialize Array(u32 0 ("element"), 0 ("dimension size")) -> (w891:u32[])
        n398 = Initialize Array(0.0 ("element"), 1024 ("dimension size"), 0 ("dimension size")) -> (w889:dbl[][])
        n399 = Bundle By Name(cluster=w892, "acq num"=w891, "signal (accum.)"=w889, "signal anis. (accum.)"=w889) -> (w890:T8)
      }
      frame "process" {
        # "!!! ONLY FIRST TRIGGER CHANNEL\nIS CHOPPER STATE, ONLY BECAME\nRELEVANT TO MA/r !!!!!!!"
        # "transfer also trig and PD"
        n400 = Tick Count (ms)() -> (millisecond timer value=w903:u32)
        n401 = Unbundle By Name(w908) -> ("raw data"=w955:dbl[][][], "trigger"=w954:bool[][], "raw PDs"=w922:dbl[][])
        n402 = Unbundle By Name(w939) -> ("acq num"=w943:u32[], "signal (accum.)"=w942:dbl[][], "signal anis. (accum.)"=w905:dbl[][], "curr acq"=w907:i32)
        n403 = feedback #1() -> (w948:u32)
        n404 = feedback-in #1(w903) -> ()
        n405 = Subtract(x=w903, y=w948) -> (x-y=→"single loop time":u32)
        n406 = for {
          tunnel: w955 -> [w1002] mode=indexing
          tunnel: w954 -> [w995]
          tunnel: [w1001] -> w914 mode=indexing
          tunnel: [w1000] -> w938 mode=indexing
          tunnel: w922 -> [w997] mode=indexing
          tunnel: [w996] -> w921 mode=indexing
          # "loop over sig. and ref."
          n407 = Index Array(array=w995) -> (element=w994:bool[])  [unwired: 2 in]
          n408 = Equal To 0?(x="parity?") -> (x = 0?=w999:bool)
          n409 = call "check_signal_chopper_state.vi"("parity?"=w999, "PD in"=w997, "chopper"=w994, "data"=w1002) -> ("PD out"=w996:dbl[], "chopper out"=w1000:bool[], "data out"=w1001:dbl[][])  [unwired: 5 in]
        }
        n410 = Array Size(array=w943) -> (size(s)=w915:i32)
        n411 = Less Or Equal?(x="history length", y=w915) -> (x <= y?=w944:bool)
        n412 = case shown="True" "use dynamic offset?" {
          tunnel: w914 -> [_ w963]
          tunnel: [w959 w962] -> w912
          frame False {
            n413 = Build Array("baseline offset (signal)", "baseline offset (ref.)") -> (w959:dbl[])
          }
          frame True {
            n414 = for {
              tunnel: w963 -> [w967] mode=indexing
              tunnel: [w965] -> w962 mode=indexing
              n415 = Index Array(array=w967, index (col)=0 ("index (row)")) -> (element=w966:dbl[])  [unwired: 1 in]
              n416 = call-poly <vilib>:"Mean.vi"("X"=w966) -> ("mean"=w965:dbl)  [unwired: 1 out]
            }
          }
        }
        "dynamic offset" <- w912
        n417 = case shown="True" w944 {
          tunnel: w943 -> [w980 w993]
          tunnel: [w980 w991] -> w940
          tunnel: w942 -> [w979 w990]
          tunnel: [w979 w989] -> w941
          tunnel: "history length" -> [_ w987]
          tunnel: w915 -> [_ w986]
          tunnel: w905 -> [w978 w983]
          tunnel: [w978 w981] -> w901
          frame False {
          }
          frame True {
            n418 = Subtract(x=w987, y=w986) -> (x-y=w985:i32)
            n419 = Absolute Value(x=w985) -> (abs(x)=w982:i32)
            n420 = Delete From Array(array=w993, length=w982, index=0) -> (array with subset deleted=w991:u32[])  [unwired: 1 out]
            n421 = Delete From Array(array=w990, length=w982, index (row)=0 ("disabled index (col)")) -> (array with subset deleted=w989:dbl[][])  [unwired: 1 in, 1 out]
            n422 = Delete From Array(array=w983, length=w982, index (row)=0 ("disabled index (col)")) -> (array with subset deleted=w981:dbl[][])  [unwired: 1 in, 1 out]
          }
        }
        n423 = Index Array(array=w938) -> (element #1=w951:bool[], element #2=w950:bool[])  [unwired: 4 in]
        n424 = for {
          tunnel: w938 -> [w977] mode=indexing
          tunnel: [w973] -> w923 mode=indexing
          n425 = Decimate 1D Array(w977) -> (w976:bool[], w975:bool[])
          n426 = Equal?(x=w976, y=w975) -> (x = y?=w974:bool[])
          n427 = Or Array Elements(Boolean array=w974) -> (logical OR=w973:bool)
        }
        "skipped" <- w923
        n428 = Exclusive Or(1:w950, 2:w951) -> (0:w946:bool[])
        n429 = Index Array(array=w914) -> (element #1=w953:dbl[][], element #2=w952:dbl[][])  [unwired: 6 in]
        n430 = Or Array Elements(Boolean array=w946) -> (logical OR=→"synchronization error":bool)
        n431 = Insert Into Array(array=w938, new element=w946) -> (→"chopper out":bool[][])  [unwired: 2 in]
        n432 = Index Array(array=w912) -> (element #1=w911:dbl, element #2=w910:dbl)  [unwired: 2 in]
        n433 = Subtract(x=w953, y=w911) -> (x-y=w909:dbl[][])
        n434 = Subtract(x=w952, y=w910) -> (x-y=w935:dbl[][])
        n435 = Insert Into Array(array=w940, new element=w907) -> (w928:u32[])  [unwired: 1 in]
        n436 = call "ta_calc_diff.vi"("data in"=w909, "ref in"=w935, "Algorithm"="Algorithm", "PD values in"=w921) -> ("pumped std"=w930:dbl[], "unpumped std"=w931:dbl[], "pumped"=w918:dbl[], "unpumped"=w932:dbl[], "diff std"=w917:dbl[], "diff"=w919:dbl[], "anisotropy"=w897:dbl[], "ref std"=w927:dbl[], "ref mean"=w925:dbl[])  [unwired: 3 in]
        n437 = Select(t=w919, s="is measurement TA?", f=w918) -> (s? t:f=w899:dbl[])
        n438 = Insert Into Array(array=w941, new element=w899) -> (w929:dbl[][])  [unwired: 2 in]
        n439 = Insert Into Array(array=w901, new element=w897) -> (w900:dbl[][])  [unwired: 2 in]
        n440 = Increment(x=w907) -> (x+1=w906:i32)
        n441 = Bundle By Name(cluster=w908, "command"=data_process."plot") -> (w934:T6)
        n442 = Bundle By Name(cluster=w939, "signal anis."=w897, "signal std"=w917, "pumped std"=w930, "unpumped std"=w931, "pumped mean"=w918, "unpumped mean"=w932, "signal"=w919, "reference mean"=w925, "reference std"=w927, "acq num"=w928, "signal (accum.)"=w929, "signal anis. (accum.)"=w900, "curr acq"=w906) -> (w926:T8)
        n443 = case shown="False" "show reference spectrum?" {
          tunnel: w926 -> [w971 w972]
          tunnel: w918 -> [w970 _]
          tunnel: w925 -> [w969 _]
          tunnel: [w968 w972] -> w904
          frame False {
            n444 = Bundle By Name(cluster=w971, "pumped stored"=w970, "reference stored"=w969) -> (w968:T8)
          }
          frame True {
          }
        }
        n445 = flat-sequence {
          tunnel: w904 -> [_]
          tunnel: w903 -> [w957]
          tunnel: [w956] -> w902
          frame #0 {
            n446 = Tick Count (ms)() -> (millisecond timer value=w958:u32)
            n447 = Subtract(x=w958, y=w957) -> (x-y=w956:u32)
          }
        }
        n448 = Enqueue Element At Opposite End(queue=w937, element=w934, error in (no error)=w936) -> ()  [unwired: 1 in, 3 out]
        "data proc." <- w902
      }
      frame "plot" {
        n449 = Unbundle By Name(w1004) -> ("pumped mean"=w1078:dbl[], "unpumped mean"=w1077:dbl[], "reference mean"=w1076:dbl[], "signal"=w1037:dbl[], "signal anis."=w1031:dbl[], "pumped stored"=w1030:dbl[], "reference stored"=w1021:dbl[])  [unwired: 1 out]
        n450 = Unbundle By Name(w1009) -> ("wavelength"=w1019:dbl[])
        n451 = Unbundle By Name(w1009) -> ("wavelength"=w1064:dbl[], "raw data"=w1063:dbl[][][], "raw PDs"=w1051:dbl[][], "trigger"=w1050:bool[][])
        n452 = Tick Count (ms)() -> (millisecond timer value=w1006:u32)
        n453 = Unbundle By Name(w1009) -> ("save flag"=w1060:bool, "save type"=w1062:bool[], "scan done?"=w1008:bool)  [unwired: 1 out]
        "scan done?" <- w1008
        n454 = Add(x=w1037, y=w1021) -> (x+y=w1038:dbl[])
        n455 = Array Size(array=w1021) -> (size(s)=w1034:i32)
        n456 = Subtract(x=w1037, y=w1021) -> (x-y=w1036:dbl[])
        n457 = Array Size(array=w1021) -> (size(s)=w1025:i32)
        n458 = Array Size(array=w1021) -> (size(s)=w1022:i32)
        n459 = Index Array(array=w1062, index=3) -> (element=w1059:bool)
        n460 = Bundle("wavelength"=w1019, "pumped mean"=w1078) -> (w1081:cluster{"wavelength":dbl[], "pumped mean":dbl[]})  [unwired: 1 in]
        n461 = Bundle("wavelength"=w1019, "unpumped mean"=w1077) -> (w1080:T15)  [unwired: 1 in]
        n462 = Bundle("wavelength"=w1019, "reference mean"=w1076) -> (w1075:T16)  [unwired: 1 in]
        n463 = Bundle("wavelength"=w1019, "signal"=w1037) -> (w1074:cluster{"wavelength":dbl[], "signal":dbl[]})  [unwired: 1 in]
        n464 = property on="main graph" class="XYGraph (strict)"() -> ("CrsrList"=w1066:T13)  [unwired: 2 in, 2 out]
        n465 = Bundle("wavelength"=w1019, "reference stored"=w1021) -> (w1029:T17)  [unwired: 1 in]
        n466 = Bundle("wavelength"=w1019, "pumped stored"=w1030) -> (w1028:T18)  [unwired: 1 in]
        n467 = Bundle("wavelength"=w1019, "signal anis."=w1031) -> (w1027:T19)  [unwired: 1 in]
        n468 = Initialize Array(0.0 ("element"), w1034) -> (w1033:dbl[])
        n469 = call "view_full_data.vi"("data"=w1063, "wavelength"=w1064) -> ()  [unwired: 10 in]
        n470 = call "error_anal.vi"("data"=w1063, "wavelength"=w1064) -> ()  [unwired: 10 in]
        n471 = Initialize Array(0.4 ("element"), w1025) -> (w1024:dbl[])
        n472 = Initialize Array(-0.2 ("element"), w1022) -> (w1020:dbl[])
        n473 = Or(x=w1060, y=w1059) -> (x .or. y?=w1014:bool)
        n474 = for {
          tunnel: w1066 -> [w1123] mode=indexing
          tunnel: w1064 -> [w1129]
          tunnel: [w1128] -> w1055 mode=indexing
          tunnel: [w1125] -> w1056 mode=indexing
          tunnel: [w1124] -> w1065 mode=indexing
          n475 = Unbundle By Name(w1123) -> ("Position.Y"=w1128:dbl, "Position.X"=w1124:dbl)
          n476 = Subtract(x=w1129, y=w1124) -> (x-y=w1127:dbl[])
          n477 = Absolute Value(x=w1127) -> (abs(x)=w1126:dbl[])
          n478 = Array Max & Min(array=w1126) -> (min index (indices)=w1125:i32)  [unwired: 3 out]
        }
        "Cursor position (idx)" <- w1056
        "Cursor position (wl)" <- w1065
        n479 = Bundle("wavelength"=w1019, w1033) -> (w1032:cluster{"wavelength":dbl[], dbl[]})  [unwired: 1 in]
        n480 = And(x=w1008, y="FROG?") -> (x .and. y?=w1013:bool)
        n481 = Bundle("wavelength"=w1019, w1038) -> (w1018:cluster{"wavelength":dbl[], dbl[]})  [unwired: 1 in]
        n482 = Bundle("wavelength"=w1019, w1036) -> (w1017:cluster{"wavelength":dbl[], dbl[]})  [unwired: 1 in]
        n483 = Bundle("wavelength"=w1019, w1024) -> (w1016:cluster{"wavelength":dbl[], dbl[]})  [unwired: 1 in]
        n484 = Bundle("wavelength"=w1019, w1020) -> (w1015:cluster{"wavelength":dbl[], dbl[]})  [unwired: 1 in]
        n485 = for {
          tunnel: [w1095] -> w1046 mode=indexing
          tunnel: [w1100] -> w1049 mode=indexing
          tunnel: i32[] [] -> [w1099]
          tunnel: dbl[] [] -> [w1098]
          tunnel: w1051 -> [w1097] mode=indexing
          tunnel: w1050 -> [w1096] mode=indexing
          tunnel: [w1094] -> w1045 mode=indexing
          tunnel: [w1090] -> w1039 mode=indexing
          n486 = for {
            shift-right: [w1102] -> w1093
            shift-left: w1098 -> [w1108]
            shift-right: [w1107] -> w1101
            shift-left: w1099 -> [w1106]
            tunnel: w1097 -> [w1104] mode=indexing
            tunnel: w1096 -> [w1103] mode=indexing
            i -> [w1105]
            n487 = case shown="True" w1103 {
              tunnel: [w1109 w1116] -> w1102
              tunnel: w1108 -> [w1109 w1115]
              tunnel: [w1110 w1114] -> w1107
              tunnel: w1106 -> [w1110 w1113]
              tunnel: w1105 -> [_ w1112]
              tunnel: w1104 -> [_ w1111]
              frame False {
              }
              frame True {
                n488 = Build Array (concatenate)(w1113, w1112) -> (w1114:i32[])
                n489 = Build Array (concatenate)(w1115, w1111) -> (w1116:dbl[])
              }
            }
          }
          n490 = call <vilib>:"Histogram.vi"("X"=w1093) -> ("X Values"=w1091:dbl[], "Histogram: h(x)"=w1092:i32[])  [unwired: 7 in, 2 out]
          n491 = Bundle(w1101, w1093) -> (w1100:cluster{i32[], dbl[]})  [unwired: 1 in]
          n492 = call <vilib>:"Std Deviation and Variance.vi"("X"=w1093) -> ("mean"=w1095:dbl, "standard deviation"=w1094:dbl)  [unwired: 1 in, 1 out]
          n493 = Bundle("Histogram: h(x)"=w1092, "X Values"=w1091) -> (w1090:T20)  [unwired: 1 in]
        }
        "PD" <- w1049
        "PD hist" <- w1039
        "PDs mean" <- w1046
        "PDs std" <- w1045
        n494 = case shown="True" w1013 {
          tunnel: w1009 -> [_ w1087]
          tunnel: w1012 -> [_ w1086]
          tunnel: w1011 -> [_ w1085]
          frame False {
          }
          frame True {
            n495 = Bundle By Name(cluster=w1087, "command"=data_process."post-processing") -> (w1088:T6)
            n496 = Enqueue Element At Opposite End(queue=w1086, element=w1088, error in (no error)=w1085) -> ()  [unwired: 1 in, 3 out]
          }
        }
        n497 = Build Array(w1081, w1080, w1075, w1074, w1027, w1028, w1029, w1032, w1016, w1015, w1018, w1017) -> (w1058:T21)
        n498 = local write "main graph"(w1058) -> ()
        n499 = Unbundle By Name(w1004) -> ("pumped std"=w1073:dbl[], "unpumped std"=w1072:dbl[], "reference std"=w1071:dbl[], "signal"=w1070:dbl[], "signal (accum.)"=w1069:dbl[][])
        n500 = Unbundle By Name(w1004) -> ("signal anis. (accum.)"=→"signal anis. (accum.)":dbl[][])
        n501 = local read "Tab Control"() -> (w1079:T2)
        n502 = case shown="\"y/x\"" w1079 {
          tunnel: w1019 -> [_ _ w1140]
          tunnel: w1073 -> [_ _ w1139]
          tunnel: w1072 -> [_ _ w1138]
          tunnel: w1071 -> [_ _ w1137]
          tunnel: w1070 -> [w1130 _ _]
          tunnel: w1069 -> [_ w1132 _]
          frame "x/y", Default {
            n503 = Build Array(w1130) -> (→"Intensity Chart":dbl[][])
          }
          frame "y/x" {
            n504 = Transpose 2D Array(2D array=w1132) -> (transposed array=w1135:dbl[][])
            n505 = Multiply(x=w1135, y=1000.0) -> (x*y=→"Intensity Graph":dbl[][])
          }
          frame "std" {
            n506 = Bundle("wavelength"=w1140, "pumped std"=w1139) -> (w1141:cluster{"wavelength":dbl[], "pumped std":dbl[]})  [unwired: 1 in]
            n507 = Bundle("wavelength"=w1140, "unpumped std"=w1138) -> (w1142:T22)  [unwired: 1 in]
            n508 = Bundle("wavelength"=w1140, "reference std"=w1137) -> (w1143:T23)  [unwired: 1 in]
            n509 = Build Array(w1141, w1142, w1143) -> (→"std graph":T24)
          }
        }
        n510 = Array To Cluster(array=w1055) -> (cluster=→"Waveform Chart":T3)
        n511 = flat-sequence {
          tunnel: w1007 -> [_]
          tunnel: w1006 -> [w1083]
          tunnel: [w1082] -> w1005
          frame #0 {
            n512 = Tick Count (ms)() -> (millisecond timer value=w1084:u32)
            n513 = Subtract(x=w1084, y=w1083) -> (x-y=w1082:u32)
          }
        }
        n514 = case shown="True" w1014 {
          tunnel: w1012 -> [_ w1120]
          tunnel: w1011 -> [_ w1119]
          tunnel: w1009 -> [_ w1118]
          frame False {
          }
          frame True {
            n515 = Bundle By Name(cluster=w1118, "command"=data_process."save") -> (w1122:T6)
            n516 = Enqueue Element At Opposite End(queue=w1120, element=w1122, error in (no error)=w1119) -> ()  [unwired: 1 in, 3 out]
          }
        }
        n517 = Unbundle By Name(w1004) -> ("acq num"=w1068:u32[])
        n518 = First Call?() -> (First Call?: T/F=w1057:bool)
        n519 = Add(x=w1046, y=w1045) -> (x+y=w1047:dbl[])
        n520 = Subtract(x=w1046, y=w1045) -> (x-y=w1007:dbl[])
        n521 = case shown="True" w1057 {
          tunnel: w1056 -> [_ _]
          frame False {
          }
          frame True {
            n522 = property on="main graph" class="XYGraph (strict)"("Cursor.Cursor X"=500.0 ("Cursor.Cursor Position:Cursor X")) -> ()  [unwired: 2 in, 2 out]
          }
        }
        n523 = Index Array(array=w1007) -> (element #1=→"Tank 1 - std" →"element 3":dbl, element #2=→"Tank 2 + std":dbl)  [unwired: 2 in]
        n524 = Index Array(array=w1046) -> (element #1=→"Tank 1" →"mean":dbl, element #2=→"Tank 2":dbl)  [unwired: 2 in]
        n525 = Index Array(array=w1047) -> (element #1=→"Tank 1 + std" →"element 2":dbl, element #2=→"Tank 2 - std":dbl)  [unwired: 2 in]
        n526 = Index Array(array=w1068) -> (element=w1067:u32)  [unwired: 1 in]
        n527 = property on="Intensity Graph" class="IntGraph (strict)"("YScale.Offset"=w1067) -> ()  [unwired: 2 in, 2 out]
        "plot time" <- w1005
      }
      frame "post-processing" {
        n528 = Unbundle By Name(w1148) -> ("scn_step_time_dly (set) [fs]"=w1146:dbl[][], "wavelength"=w1147:dbl[])
        n529 = Unbundle By Name(w1150) -> ("signal (accum.)"=w1149:dbl[][])
        n530 = Index Array(array=w1146) -> (element=w1145:dbl[])  [unwired: 2 in]
        n531 = call "FROG.vi"("wl_min_max"="FROG wl_min_max", "data"=w1149, "wl"=w1147, "time"=w1145) -> ()  [unwired: 8 in]
      }
      frame "save" {
        # "this won't work atm"
        n532 = Unbundle By Name(w1153) -> ("scn_step_time_dly (set) [fs]"=w1155:dbl[][], "scn_step"=w1177:i32, "save type"=w1172:bool[], "scn_iter"=w1178:i32, "wavelength"=w1183:dbl[], "raw data"=w1179:dbl[][][], "scn_step_time_dly (set) [fs]"=w1154:dbl[][], "save path"=w1174:path)  [unwired: 1 out]
        n533 = Unbundle By Name(w1152) -> ("pumped mean"=w1182:dbl[], "unpumped mean"=w1181:dbl[], "reference mean"=w1180:dbl[], "signal (accum.)"=w1175:dbl[][], "signal anis. (accum.)"=w1151:dbl[][])
        n534 = Increment(x=w1177) -> (x+1=w1157:i32)
        n535 = Array Size(array=w1155) -> (size(s)=w1161:i32[])
        n536 = Index Array(array=w1155) -> (element=w1164:dbl[])  [unwired: 2 in]
        n537 = Build Array("Title", "Experimenter", "Experimental parameters") -> (w1165:string[])
        n538 = Index Array(array=w1161) -> (element=w1159:i32)  [unwired: 1 in]
        n539 = Array Size(array=w1164) -> (size(s)=w1176:i32)
        n540 = Index Array(array=w1172, index=3) -> (element=w1171:bool)
        n541 = Decrement(x=w1159) -> (x-1=w1160:i32)
        n542 = Equal?(x=w1176, y=w1157) -> (x = y?=w1173:bool)
        n543 = Index Array(array=w1155, index (row)=w1160) -> (element=w1163:dbl[])  [unwired: 1 in]
        n544 = Or(x=w1173, y=w1171) -> (x .or. y?=w1169:bool)
        n545 = call "Remove Duplicates From 1D Array.vim"("array"=w1163) -> ("array with duplicates removed"=w1162:dbl[])  [unwired: 10 in]
        n546 = Array Size(array=w1162) -> (size(s)=w1158:i32)
        "size of dependent time scan 2" <- w1158
        n547 = case shown="True" w1169 {
          tunnel: w1183 -> [_ w1204]
          tunnel: w1182 -> [_ w1194]
          tunnel: w1181 -> [_ _]
          tunnel: w1180 -> [_ w1193]
          tunnel: w1179 -> [_ w1195]
          tunnel: w1172 -> [_ w1196]
          tunnel: w1178 -> [_ _]
          tunnel: w1175 -> [_ w1203]
          tunnel: w1174 -> [_ w1192]
          tunnel: w1154 -> [_ w1202]
          tunnel: w1165 -> [_ w1191]
          tunnel: w1151 -> [_ w1185]
          frame False {
          }
          frame True {
            # "crop to only the transients of current scan"
            n548 = Index Array(array=w1202) -> (element=w1186:dbl[])  [unwired: 2 in]
            n549 = Array Size(array=w1185) -> (size(s)=w1190:i32[])
            n550 = Array Size(array=w1203) -> (size(s)=w1201:i32[])
            n551 = Array Size(array=w1186) -> (size(s)=w1187:i32)
            n552 = Index Array(array=w1190) -> (element=w1189:i32)  [unwired: 1 in]
            n553 = Array Size(array=w1186) -> (size(s)=w1198:i32)
            n554 = Index Array(array=w1201) -> (element=w1200:i32)  [unwired: 1 in]
            n555 = Subtract(x=w1189, y=w1187) -> (x-y=w1188:i32)
            n556 = Subtract(x=w1200, y=w1198) -> (x-y=w1199:i32)
            n557 = Array Subset(array=w1185, index (row)=w1188, length (row)=w1187) -> (w1184:dbl[][])  [unwired: 2 in]
            n558 = Array Subset(array=w1203, index (row)=w1199, length (row)=w1198) -> (w1197:dbl[][])  [unwired: 2 in]
            n559 = call "saving.vi"("file path (use dialog)"=w1192, "save type"=w1196, "details"=w1191, "signal mean"=w1194, "wavelength"=w1204, "signal anis (accum.)"=w1184, "time delays"=w1202, "signal (accum.)"=w1197, "raw data"=w1195, "reference mean"=w1193) -> ()  [unwired: 6 in]
          }
        }
        n560 = Equal?(x=w1158, y=w1157) -> (x = y?=→"x = y?":bool)
      }
      frame "exit" {
        n561 = Release Queue(queue=w1205) -> ()  [unwired: 2 in, 3 out]
      }
    }
  }
  n562 = while {
    tunnel: w62 -> [w1212]
    tunnel: w61 -> [w1211]
    tunnel: w63 -> [w1208]
    stop <- w1210 stop-if-true
    # "Control"
    n563 = event shown="[2] \"get_single_acq\": Value Change" {
      selector: _ -> [_ _ _ _ _ _ _ _ _ _ _ _ _ _ _ _ _ _ _ _ _ _ _ _ _ _ _]
      dyn-events: _ -> [_ _ _ _ _ _ _ _ _ _ _ _ _ _ _ _ _ _ _ _ _ _ _ _ _ _ _]
      timeout: 10 -> [_ _ _ _ _ _ _ _ _ _ _ _ _ _ _ _ _ _ _ _ _ _ _ _ _ _ _]
      tunnel: w1212 -> [_ w1231 w1252 w1256 w1270 w1280 _ _ _ _ _ w1317 w1328 _ _ w1347 w1362 w1368 w1383 _ w1392 w1397 _ _ _ _ w1436]
      tunnel: w1211 -> [_ w1230 w1251 w1255 w1269 w1279 _ _ _ _ _ w1318 w1327 _ _ w1346 w1361 w1367 w1382 _ w1391 w1396 _ _ _ _ w1435]
      tunnel: [_ _ _ _ _ _ _ _ _ _ _ _ _ _ _ _ _ _ _ _ _ _ _ _ _ _ w1437] -> w1210
      tunnel: w1208 -> [_ w1232 w1250 w1253 w1267 w1278 _ _ _ _ _ w1316 w1326 _ _ w1348 w1360 w1370 w1384 _ w1389 w1398 _ _ _ _ w1434]
      event Timeout {
        n564 = event-data() -> ()  [unwired: 1 in, 3 out]
        n565 = local read "is measurement TA?"() -> (w1213:bool)
        n566 = case shown="False" w1213 {
          tunnel: [w1218 w1226] -> w1215
          tunnel: [w1217 w1225] -> w1214
          frame False {
            w1219 = 1000.0 ("y")
            n567 = local read "ampl"() -> (w1224:cluster{dbl, dbl})
            n568 = Unbundle(w1224) -> (w1221:dbl, w1223:dbl)
            n569 = Multiply(x=w1221, y=w1219) -> (x*y=w1220:dbl)
            n570 = Multiply(x=w1223, y=w1219) -> (x*y=w1222:dbl)
            n571 = Max & Min(x=w1220, y=w1222) -> (max(x,y)=w1218:dbl, min(x,y)=w1217:dbl)
          }
          frame True {
            n572 = Divide(x="diff", y=1.0) -> (x/y=w1226:dbl)
            n573 = Negate(x=w1226) -> (-x=w1225:dbl)
          }
        }
        n574 = property on="main graph" class="XYGraph (strict)"("ActYScl"=1 ("Active Y Scale"), "YScale.Maximum"=w1215, "YScale.Minimum"=w1214) -> ()  [unwired: 2 in, 2 out]
        n575 = property on="Intensity Chart" class="IntChart (strict)"("ZScale.Maximum"=w1215, "ZScale.Minimum"=w1214) -> ()  [unwired: 2 in, 2 out]
        n576 = property on="Intensity Graph" class="IntGraph (strict)"("ZScale.Maximum"=w1215, "ZScale.Minimum"=w1214) -> ()  [unwired: 2 in, 2 out]
      }
      event "calibrate wavelength": Value Change {
        n577 = event-data() -> ("NewVal"=w1229:bool)  [unwired: 1 in]
        n578 = case shown="False" w1229 {
          tunnel: w1232 -> [w1235 w1244]
          tunnel: w1231 -> [w1234 w1243]
          tunnel: w1230 -> [w1233 w1242]
          frame False {
            n579 = To Variant(anything=FALSE) -> (Variant=w1236:variant)
            n580 = Bundle(cluster=w1235, "state"=state."cam_set_wl" ("element"), "value"=w1236) -> (w1238:cluster{"state":T7, "value":variant})
            n581 = Enqueue Element(queue=w1234, element=w1238, error in (no error)=w1233) -> ()  [unwired: 1 in, 3 out]
          }
          frame True {
            n582 = To Variant(anything=TRUE) -> (Variant=w1240:variant)
            n583 = Bundle(cluster=w1244, "state"=state."cam_set_wl" ("element"), "value"=w1240) -> (w1245:cluster{"state":T7, "value":variant})
            n584 = Enqueue Element(queue=w1243, element=w1245, error in (no error)=w1242) -> ()  [unwired: 1 in, 3 out]
          }
        }
      }
      event "get_single_acq": Value Change {
        n585 = event-data() -> ("OldVal"=w1248:bool)  [unwired: 1 in]
        n586 = Bundle(cluster=w1250, "state"=state."cam_single_acq") -> (w1249:cluster{"state":T7, "value":variant})  [unwired: 1 in]
        n587 = Enqueue Element(queue=w1252, element=w1249, error in (no error)=w1251) -> ()  [unwired: 1 in, 3 out]
        n588 = property on="get_single_acq" class="Bool (strict)"("Value"=w1248) -> ()  [unwired: 2 in, 2 out]
      }
      event "get bg": Value Change {
        n589 = event-data() -> ("NewVal"=w1254:bool)  [unwired: 1 in]
        n590 = case shown="True" w1254 {
          tunnel: w1256 -> [w1261 w1266]
          tunnel: w1255 -> [w1260 w1265]
          tunnel: w1253 -> [w1259 w1264]
          frame False {
            n591 = Bundle(cluster=w1259, "state"=state."cam_rst_bg") -> (w1258:cluster{"state":T7, "value":variant})  [unwired: 1 in]
            n592 = Enqueue Element(queue=w1261, element=w1258, error in (no error)=w1260) -> ()  [unwired: 1 in, 3 out]
          }
          frame True {
            n593 = Bundle(cluster=w1264, "state"=state."cam_get_bg" ("element")) -> (w1262:cluster{"state":T7, "value":variant})  [unwired: 1 in]
            n594 = Enqueue Element(queue=w1266, element=w1262, error in (no error)=w1265) -> ()  [unwired: 1 in, 3 out]
          }
        }
      }
      event "cont acq": Value Change {
        n595 = event-data() -> ("NewVal"=w1268:bool)  [unwired: 1 in]
        n596 = case shown="True" w1268 {
          tunnel: w1270 -> [w1272 w1277]
          tunnel: w1269 -> [w1271 w1276]
          tunnel: w1267 -> [_ w1275]
          frame False {
            n597 = Flush Queue(queue=w1272, error in (no error)=w1271) -> ()  [unwired: 3 out]
          }
          frame True {
            n598 = Bundle(cluster=w1275, "state"=state."cam_cnt_acq") -> (w1274:cluster{"state":T7, "value":variant})  [unwired: 1 in]
            n599 = Enqueue Element(queue=w1277, element=w1274, error in (no error)=w1276) -> ()  [unwired: 1 in, 3 out]
          }
        }
      }
      event "center cursor": Value Change {
        n600 = event-data() -> ()  [unwired: 1 in, 2 out]
        n601 = Bundle(cluster=w1278, "state"=state."aux_center_cursor") -> (w1282:cluster{"state":T7, "value":variant})  [unwired: 1 in]
        n602 = Enqueue Element(queue=w1280, element=w1282, error in (no error)=w1279) -> ()  [unwired: 1 in, 3 out]
      }
      event "add cursor": Value Change {
        n603 = event-data() -> ()  [unwired: 1 in, 1 out]
        n604 = property on="main graph" class="XYGraph (strict)"() -> ("CrsrList"=w1290:T13)  [unwired: 2 in, 2 out]
        n605 = Array Size(array=w1290) -> (size(s)=w1284:i32)
        n606 = Index Array(array=w1290) -> (element=w1289:T14)  [unwired: 1 in]
        n607 = Index Array(array=u32[] [16776722, 16711680, 6618880, 16860, 12124158], index=w1284) -> (element=w1286:u32)
        n608 = Bundle By Name(cluster=w1289, "Color"=w1286) -> (w1288:T14)
        n609 = Insert Into Array(array=w1290, index=w1284, new element=w1288) -> (w1291:T13)
        n610 = property on="Waveform Chart" class="WFChart (strict)"("Active Plot"=w1284, "Plot.Visible?"=TRUE ("Plot.Visible")) -> ()  [unwired: 2 in, 2 out]
        n611 = property on="main graph" class="XYGraph (strict)"("CrsrList"=w1291, "Active Cursor"=w1284, "Cursor.LineWidth"=u8 2 ("Cursor.Line Width")) -> ()  [unwired: 2 in, 2 out]
      }
      event "remove cursor": Value Change {
        n612 = event-data() -> ()  [unwired: 1 in, 6 out]
        n613 = property on="main graph" class="XYGraph (strict)"() -> ("CrsrList"=w1295:T13)  [unwired: 2 in, 2 out]
        n614 = Array Size(array=w1295) -> (size(s)=w1294:i32)
        n615 = Greater?(x=w1294, y=1) -> (0:w1292:bool)
        n616 = case shown="True" w1292 {
          tunnel: w1295 -> [_ w1300]
          tunnel: w1294 -> [_ w1298]
          frame False {
          }
          frame True {
            n617 = Decrement(x=w1298) -> (x-1=w1296:i32)
            n618 = Delete From Array(array=w1300, index=w1296) -> (array with subset deleted=w1299:T13)  [unwired: 1 in, 1 out]
            n619 = property on="Waveform Chart" class="WFChart (strict)"("Active Plot"=w1296, "Plot.Visible?"=FALSE ("Plot.Visible")) -> ()  [unwired: 2 in, 2 out]
            n620 = property on="main graph" class="XYGraph (strict)"("CrsrList"=w1299) -> ()  [unwired: 2 in, 2 out]
          }
        }
      }
      event "camera max scale": Value Change {
        n621 = event-data() -> ("NewVal"=w1301:u16)  [unwired: 1 in]
        n622 = case shown="2" w1301 {
          tunnel: [65.535 16.384 4.096] -> w1302
          frame 0, Default {
          }
          frame 1 {
          }
          frame 2 {
          }
        }
        n623 = property on="ampl" class="Slide (strict)"("Scale.Maximum"=w1302) -> ()  [unwired: 2 in, 2 out]
      }
      event "ampl": Value Change {
        w1307 = 1000.0 ("y")
        n624 = event-data() -> ()  [unwired: 1 in, 6 out]
        n625 = Unbundle("ampl") -> (w1309:dbl, w1311:dbl)
        n626 = Multiply(x=w1309, y=w1307) -> (x*y=w1308:dbl)
        n627 = Multiply(x=w1311, y=w1307) -> (x*y=w1310:dbl)
        n628 = Max & Min(x=w1308, y=w1310) -> (max(x,y)=w1313:dbl, min(x,y)=w1312:dbl)
        n629 = property on="main graph" class="XYGraph (strict)"("ActYScl"=0 ("Active Y Scale"), "YScale.Maximum"=w1313, "YScale.Minimum"=w1312) -> ()  [unwired: 2 in, 2 out]
      }
      event "Scale.Range:Maximum": Value Change {
        n630 = event-data() -> ("NewVal"=w1315:dbl)  [unwired: 1 in, 5 out]
        n631 = property on="diff" class="Slide (strict)"("Scale.Maximum"=w1315) -> ()  [unwired: 2 in, 2 out]
      }
      event "save wl calibration to .ini": Value Change {
        n632 = event-data() -> ("OldVal"=w1321:bool)  [unwired: 1 in]
        n633 = Bundle(cluster=w1316, "state"=state."aux_save_wl_to_ini") -> (w1320:cluster{"state":T7, "value":variant})  [unwired: 1 in]
        n634 = Enqueue Element(queue=w1317, element=w1320, error in (no error)=w1318) -> ()  [unwired: 1 in, 3 out]
        n635 = property on="save wl calibration to .ini" class="Bool (strict)"("Value"=w1321) -> ()  [unwired: 2 in, 2 out]
      }
      event "stage position(s)": Value Change {
        n636 = event-data() -> ("NewVal"=w1322:dbl[])  [unwired: 1 in]
        n637 = To Variant(anything=w1322) -> (Variant=w1323:variant)
        n638 = Bundle(cluster=w1326, "state"=state."stg_set_pos", "value"=w1323) -> (w1325:cluster{"state":T7, "value":variant})
        n639 = Enqueue Element(queue=w1328, element=w1325, error in (no error)=w1327) -> ()  [unwired: 1 in, 3 out]
      }
      event "set as t0": Value Change {
        n640 = event-data() -> ("NewVal"=w1337:bool[], "OldVal"=w1329:bool[])  [unwired: 1 in]
        n641 = for {
          tunnel: w1337 -> [w1342] mode=indexing
          tunnel: w1329 -> [w1340]
          tunnel: [w1341] -> w1336 mode=indexing
          i -> [w1339]
          n642 = Index Array(array=w1340, index=w1339) -> (element=w1338:bool)
          n643 = Not Equal?(x=w1342, y=w1338) -> (x != y?=w1341:bool)
        }
        n644 = property on="stage position(s)" class="Arr (strict)"() -> ("Value"=w1332:dbl[])  [unwired: 2 in, 2 out]
        n645 = local write "set as t0"(w1329) -> ()
        n646 = Search 1D Array(1D array=w1336, element=TRUE) -> (index of element=w1331:i32)  [unwired: 1 in]
        n647 = Index Array(array=w1332, index=w1331) -> (element=w1330:dbl)
        n648 = Replace Array Subset(array="t0 position(s)", new element=w1330, index=w1331) -> (w1334:dbl[])
        n649 = property on="t0 position(s)" class="Arr (strict)"("Value"=w1334) -> ()  [unwired: 2 in, 2 out]
      }
      event "t0 position(s)": Value Change {
        n650 = event-data() -> ()  [unwired: 1 in, 6 out]
      }
      event "home stages": Value Change {
        # "find out which stage to home"
        n651 = event-data() -> ("NewVal"=w1345:bool[], "OldVal"=w1344:bool[])  [unwired: 1 in]
        n652 = for {
          tunnel: w1345 -> [w1357] mode=indexing
          tunnel: w1344 -> [w1355]
          tunnel: [w1356] -> w1352 mode=indexing
          i -> [w1354]
          n653 = Index Array(array=w1355, index=w1354) -> (element=w1353:bool)
          n654 = Not Equal?(x=w1357, y=w1353) -> (x != y?=w1356:bool)
        }
        n655 = Search 1D Array(1D array=w1352, element=TRUE) -> (index of element=w1349:i32)  [unwired: 1 in]
        n656 = Bundle(cluster=w1348, "state"=state."stg_home", "value"=w1349) -> (w1350:cluster{"state":T7, "value":variant})
        n657 = Enqueue Element(queue=w1347, element=w1350, error in (no error)=w1346) -> ()  [unwired: 1 in, 3 out]
      }
      event "time delay file": Value Change {
        n658 = event-data() -> ("NewVal"=w1359:path)  [unwired: 1 in]
        n659 = To Variant(anything=w1359) -> (Variant=w1358:variant)
        n660 = Bundle(cluster=w1360, "state"=state."scn_load_step_file", "value"=w1358) -> (w1364:cluster{"state":T7, "value":variant})
        n661 = Enqueue Element(queue=w1362, element=w1364, error in (no error)=w1361) -> ()  [unwired: 1 in, 3 out]
      }
      event "scan": Value Change {
        n662 = event-data() -> ("NewVal"=w1369:bool)  [unwired: 1 in]
        n663 = Flush Queue(queue=w1368, error in (no error)=w1367) -> (queue out=w1365:refnum<queue>, error out=w1366:errorcluster)  [unwired: 1 out]
        n664 = case shown="False" w1369 {
          tunnel: w1365 -> [_ w1372]
          tunnel: w1366 -> [_ w1371]
          tunnel: w1370 -> [_ w1377]
          frame False {
          }
          frame True {
            w1375 = 0
            n665 = Build Array(w1375, w1375) -> (w1374:i32[])
            n666 = To Variant(anything=w1374) -> (Variant=w1373:variant)
            n667 = Bundle(cluster=w1377, "state"=state."scn_init", "value"=w1373) -> (w1378:cluster{"state":T7, "value":variant})
            n668 = Enqueue Element(queue=w1372, element=w1378, error in (no error)=w1371) -> ()  [unwired: 1 in, 3 out]
          }
        }
      }
      event "save type": Value Change {
        n669 = event-data() -> ("NewVal"=w1379:bool[])  [unwired: 1 in]
        n670 = To Variant(anything=w1379) -> (Variant=w1381:variant)
        n671 = Bundle(cluster=w1384, "state"=state."dat_update_save_type", "value"=w1381) -> (w1385:cluster{"state":T7, "value":variant})
        n672 = Enqueue Element(queue=w1383, element=w1385, error in (no error)=w1382) -> ()  [unwired: 1 in, 3 out]
      }
      event "index": Value Change {
        n673 = event-data() -> ()  [unwired: 1 in, 2 out]
        n674 = Build Array("index") -> (w1386:u16[])
        n675 = property on="pixel/index" class="Arr (strict)"("Index Values"=w1386) -> ()  [unwired: 2 in, 2 out]
        n676 = property on="wavelength \n(calibration value)" class="Arr (strict)"("Index Values"=w1386) -> ()  [unwired: 2 in, 2 out]
        n677 = property on="wavelength (fitted)" class="Arr (strict)"("Index Values"=w1386) -> ()  [unwired: 2 in, 2 out]
      }
      event "save raw data": Value Change {
        n678 = event-data() -> ("OldVal"=w1393:bool)  [unwired: 1 in]
        n679 = Bundle(cluster=w1389, "state"=state."dat_save_raw") -> (w1388:cluster{"state":T7, "value":variant})  [unwired: 1 in]
        n680 = property on="save raw data" class="Bool (strict)"("Value"=w1393) -> ()  [unwired: 2 in, 2 out]
        n681 = Enqueue Element(queue=w1392, element=w1388, error in (no error)=w1391) -> ()  [unwired: 1 in, 3 out]
      }
      event "save flag": Value Change {
        n682 = event-data() -> ("NewVal"=w1395:bool)  [unwired: 1 in]
        n683 = To Variant(anything=w1395) -> (Variant=w1399:variant)
        n684 = Bundle(cluster=w1398, "state"=state."dat_update_save_flag", "value"=w1399) -> (w1400:cluster{"state":T7, "value":variant})
        n685 = Enqueue Element(queue=w1397, element=w1400, error in (no error)=w1396) -> ()  [unwired: 1 in, 3 out]
      }
      event "view error anal": Value Change {
        n686 = event-data() -> ("NewVal"=w1402:bool)  [unwired: 1 in]
        n687 = vi-ref "error_anal.vi"() -> (w1401:refnum<vi>)
        n688 = case shown="False" w1402 {
          tunnel: w1401 -> [w1407 w1410]
          tunnel: [w1405 w1409] -> w1403
          tunnel: [w1406 w1408] -> w1404
          frame False {
            n689 = invoke class="VI" method="FP.Close"(reference=w1407) -> (reference out=w1406:refnum<vi>, error out=w1405:errorcluster)  [unwired: 2 in, 1 out]
          }
          frame True {
            n690 = invoke class="VI" method="FP.Open"(reference=w1410) -> (reference out=w1408:refnum<vi>, error out=w1409:errorcluster)  [unwired: 4 in, 3 out]
          }
        }
        n691 = Close Reference(reference=w1404, error in (no error)=w1403) -> ()  [unwired: 1 out]
      }
      event "view full data": Value Change {
        n692 = event-data() -> ("NewVal"=w1414:bool)  [unwired: 1 in]
        n693 = vi-ref "view_full_data.vi"() -> (w1413:refnum<vi>)
        n694 = case shown="True" w1414 {
          tunnel: w1413 -> [w1417 w1420]
          tunnel: [w1415 w1419] -> w1411
          tunnel: [w1416 w1418] -> w1412
          frame False {
            n695 = invoke class="VI" method="FP.Close"(reference=w1417) -> (reference out=w1416:refnum<vi>, error out=w1415:errorcluster)  [unwired: 2 in, 1 out]
          }
          frame True {
            n696 = invoke class="VI" method="FP.Open"(reference=w1420) -> (reference out=w1418:refnum<vi>, error out=w1419:errorcluster)  [unwired: 4 in, 3 out]
          }
        }
        n697 = Close Reference(reference=w1412, error in (no error)=w1411) -> ()  [unwired: 1 out]
      }
      event "ts_plot_lin-log": Value Change {
        n698 = event-data() -> ("NewVal"=w1422:bool)  [unwired: 1 in, 5 out]
        n699 = Boolean To (0,1)(Boolean=w1422) -> (0, 1=w1421:i16)
        n700 = property on="Waveform Graph" class="WFGraph (strict)"("YScale.Mapping Mode"=w1421) -> ()  [unwired: 2 in, 2 out]
      }
      event Key Down {
        n701 = event-data() -> ("Char"=w1424:i16)  [unwired: 1 in, 9 out]
        "Char" <- w1424
        n702 = disable-structure shown="Disabled" {
          disable-tunnel: w1424 -> [w1425 _]
          frame Disabled {
            n703 = case shown="49" w1425 {
              frame 0, Default {
              }
              frame 49 {
                n704 = property on="stage position(s)" class="Arr (strict)"("Array Element.Key Focus"=TRUE) -> ()  [unwired: 2 in, 2 out]
              }
              frame 98 {
                n705 = property on="get bg" class="Bool (strict)"() -> ("Value"=w1428:bool)  [unwired: 2 in, 2 out]
                n706 = Not(x=w1428) -> (.not. x?=w1427:bool)
                n707 = property on="get bg" class="Bool (strict)"("Val(Sgnl)"=w1427) -> ()  [unwired: 2 in, 2 out]
              }
              frame 99 {
                n708 = property on="cont acq" class="Bool (strict)"() -> ("Value"=w1430:bool)  [unwired: 2 in, 2 out]
                n709 = Not(x=w1430) -> (.not. x?=w1429:bool)
                n710 = property on="cont acq" class="Bool (strict)"("Val(Sgnl)"=w1429) -> ()  [unwired: 2 in, 2 out]
              }
              frame 115 {
                n711 = property on="get_single_acq" class="Bool (strict)"("Val(Sgnl)"=TRUE ("Value (Signaling)")) -> ()  [unwired: 2 in, 2 out]
              }
            }
          }
          frame Enabled {
          }
        }
        n712 = Wait (ms)(milliseconds to wait=u32 75) -> ()  [unwired: 1 out]
      }
      event Panel Close? {
        w1437 = TRUE
        n713 = event-data() -> ()  [unwired: 1 in, 4 out]
        n714 = Bundle(cluster=w1434, "state"=state."stop" ("element")) -> (w1432:cluster{"state":T7, "value":variant})  [unwired: 1 in]
        n715 = Enqueue Element(queue=w1436, element=w1432, error in (no error)=w1435) -> ()  [unwired: 1 in, 3 out]
        n716 = event-data("Discard?"=w1437) -> ()  [unwired: 1 in, 1 out]
      }
    }
  }
  n717 = call <vilib>:"Simple Error Handler.vi"("error in (no error)"=w93) -> ()  [unwired: 4 in, 5 out]
